vi "slow_control_2_08.vi"() -> ()   [LabVIEW 2018]
uses:
  fa57f61f-0bb9-49ac-92eb-fcb40add4dbb.vi
  499f9cf5-7b15-41ea-951a-8da9be12721d.vi
  <vilib>/DAQmx/read.llb/DAQmx Read (Analog 1D DBL NChan 1Samp).vi
  ffb0d1b3-ef19-4e2e-b36e-7277177ef4b3.vi
  9a1acc8a-69db-4048-9e4c-bb07d66d2422.vi
  <vilib>/DAQmx/create/channels.llb/DAQmx Create Channel (AI-Voltage-Basic).vi
  <vilib>/DAQmx/create/channels.llb/DAQmx Create Channel (AI-Current-Basic).vi
  <vilib>/DAQmx/create/channels.llb/DAQmx Create Channel (AI-Temperature-RTD).vi
  <vilib>/DAQmx/miscellaneous.llb/DAQmx Fill In Error Info.vi
  <vilib>/Utility/file.llb/Read Delimited Spreadsheet (string).vi
  <instrlib>/Lake Shore 335/Lake Shore 335.lvlib
  <instrlib>/CAEN PSM/CAEN PSM.lvlib
  <resource>/objmgr/daqmx.rc
panel:
  out "Cycle number":i32
  out "Alarm state":bool
  out "Timestamp last \nmeasured (UPS)":timestamp
  out "Auto-clear":bool
  in  "Auto-clear data?":bool
  in  "Clear data":bool
  in  "Clear data every N cycles":dbl
  in  "N samples":i32=30
  out "Average Flow (SLPM)":dbl caption="Flow (SLPM)"
  out "CAEN Ch. Names":string[](array[string])
  out "Heater":dbl
  out "Coldhead":dbl
  in  "Cycles to execute":dbl=5.0 format="%#_13g"
  out "Detector Pressure":dbl
  in  "N samples":i32=20
  in  "Allows tabs on \nfront panel":T1(tab)
  in  "OK Button":bool
  in  "Specify up to six temperature sensors inside \nthe detector, separated with a comma.\nNumbers only, single commas!":string="10,11,12,13,14,15"
  out "Valid example:":string="11,12, 13, 15 ,14 "
  in  "Anode ch.":enum16{"1", "2", "3", "4"}(ring)=enum."3"
  in  "CAEN unit selector":enum16{"CAEN 1", "CAEN 2"}(ring)
  in  "Multipliers":dbl[](array[numeric])=[1.0, 1.0, 1.0, 1.0, 1.0, 1.0, 1.0, 1.0]
  in  "Offsets\nsubtracted":dbl[](array[numeric])=[0.0, 0.0, 0.0, 0.0, 0.0, 0.0, 0.0, 0.0]
  in  "Channel Names (9207, ai8:15)":string[](array[string])=["i0", "i1", "i2", "i3", "i4", "i5", "i6", "i7"] caption="\"Other\""
  in  "Flow meter input:":T2(ring)=enum."v3"
  in  "Detector pressure input:":T2(ring)
  in  "Channel Names (9207, ai0:7)":string[](array[string])=["v0", "v1", "v2", "v3", "v4", "v5", "v6", "v7"] caption="\"Other\""
  in  "Multipliers":dbl[](array[numeric])=[0.2, 1.0, 1.0, 28.409091, 1.0, 1.0, 1.0, 1.0]
  in  "Offsets\nsubtracted":dbl[](array[numeric])=[0.002, 0.0, 0.0, 0.44376, 0.0, 0.0, 0.0, 0.0]
  in  "Voltage channels":tag[](array[tag])=["9207/ai0", "9207/ai1", "9207/ai2", "9207/ai3", "9207/ai4", "9207/ai5", "9207/ai6", "9207/ai7"]
  in  "COM-port CAEN 1":refnum<visa-resource-name>
  in  "COM-port CAEN 2":refnum<visa-resource-name>
  out "Temp B":dbl
  out "Temp A":dbl
  out "LakeShore readings 2":dbl[](array[numeric])
  in  "Run lakeshore?":bool
  in  "ID Query":bool
  in  "COM-port LakeShore":refnum<visa-resource-name>
  in  "PID settings":cluster{"P":dbl, "I":dbl, "D":dbl}={"P"=50.0, "I"=20.0, "D"=120.0}
  in  "Setpoint (°C)":dbl=-100.0 format="%.1f"
  in  "Heater range":u16(ring) items=["Off", "Low (On)", "Medium", "High"]
  in  "Current channels":tag[](array[tag])=["9207/ai8", "9207/ai9", "9207/ai10", "9207/ai11", "9207/ai12", "9207/ai13", "9207/ai14", "9207/ai15"]
  in  "Channel Names (CAEN)":string[](array[string])=["PMT 1", "PMT 2", "Anode", "Cathode", "Top gate", "Bottom gate", "Other 1", "Other 2"]
  in  "RTD Type":i32(ring)=12481 items=["Pt3750"=12481, "Pt3851"=10071, "Pt3911"=12482, "Pt3916"=10069, "Pt3920"=10053, "Pt3928"=12483, "Custom"=10137]
  in  "Module 1 channels (slot 1)":tag[](array[tag])
  in  "Current Excitation Source":i32(ring)=10200 items=["Internal"=10200, "External"=10167, "None"=10230]
  in  "Resistance Configuration":i32(ring)=3 items=["2-Wire"=2, "3-Wire"=3, "4-Wire"=4]
  in  "R (T = 0°C):":dbl=100.0
  in  "B":dbl
  in  "A":dbl
  in  "C":dbl
  in  "Module 2 channels (slot 2)":tag[](array[tag])
  in  "Shut off heater \nif Alarm is active":bool=TRUE
  out "Det. T.":i32[](array[numeric])
  out "9207 (V; A) Converted":dbl[](array[numeric])
  out "9216 #1 (°C)":dbl[](array[numeric])
  out "9216 #2 (°C)":dbl[](array[numeric])
  out "Raw readouts (V, mA)":dbl[](array[numeric]) format="%0.2f"
  out "Det.P input #":i32
  out "Flow input #":i32
  out "Temperatures":dbl[](array[numeric]) format="%0.2f"
  in  "Number of Bonus lines":i32=1
  out "Names (optional)":string[](array[string])
  in  "Send daily email?":bool
  in  "Phone numbers":string[](array[string])
  out "Alarm (or test) message":string
  in  "Alarm armed":bool
  in  "Repeat Alarm SMS\nevery N minutes":dbl=15.0
  in  "Test alarm":bool
  out "Warning":bool
  in  "UPS":bool
  in  "UPS Voltage \nLower Threshold":dbl=220.0
  out "String 6":string
  out "String 5":string
  out "String 4":string
  out "String 3":string
  out "String 2":string
  out "String":string
  out "NI mod 2&3 status":bool
  in  "NI mod 2&3":bool
  in  "NI mod 1":bool
  in  "CAEN 2":bool
  in  "CAEN 1":bool
  in  "LakeShore":bool
  out "Det. P. warning":bool
  out "Boolean 6":bool
  out "Boolean 5":bool
  out "Boolean 4":bool
  out "Boolean 3":bool
  out "Boolean 2":bool
  out "Boolean":bool
  in  "T 6":bool
  in  "T 5":bool
  in  "T 4":bool
  in  "T 3":bool
  in  "T 2":bool
  in  "T 1":bool
  in  "Detector Pressure":bool
  in  "Overpressure threshold":dbl
  in  "Underpressure threshold":dbl
  out "Comm. status":bool
  in  "High Temp threshold":dbl format="%#_13g"
  in  "Low Temp threshold":dbl format="%#_13g"
  out "LakeShore status":bool
  out "NI mod1 (P) status":bool
  out "CAEN 1 status":bool
  out "CAEN 2 status":bool
  out "Initialization status":bool
  out "Minimum input voltage measured":dbl
  out "Alarm active 2":bool
  out "standard error (SMS script)":string
  out "Status email preview":string
  in  "Send status email at time:":string
  in  "Email Adresses":string[](array[string])
  in  "return address":string="xamsups@gmail.com"
  in  "Ignore Initialization Errors":bool=TRUE caption="Ignore init. errors?"
  out "9207 (ai 8:15, Amperes)":cluster{timestamp[], dbl[]}[](graph)
  in  "Temperature channel selector":u16(ring)=10 items=["10"=10, "11"=11, "12"=12, "13"=13, "14"=14, "15"=15, "Average"=666]
  out "Heater power (%)":cluster{timestamp[], dbl[]}[](graph)
  out "Flow (SLPM)":cluster{timestamp[], dbl[]}[](graph)
  out "9207 (ai 0:7, Volts)":cluster{timestamp[], dbl[]}[](graph)
  out "Phase Diagram":cluster{"X":dbl, "Y":dbl}[](graph)
  out "Temperature (ai 0:15, °C)":cluster{timestamp[], dbl[]}[](graph)
  in  "Pause?":bool
  out "Integrated Flow (SL)":dbl
  in  "Reset?":bool
  out "LakeShore readings":dbl[](array[numeric])
  in  "Temperature Channel Selector":u16(ring) items=["10"=10, "11"=11, "12"=12, "13"=13, "14"=14, "15"=15]
  out "Historical Large Phase Diagram":cluster{dbl[], dbl[]}[](graph)
  out "Large Phase Diagram":cluster{"X":dbl, "Y":dbl}[](graph)
  in  "Temperature Channel Selector":u16(ring)=666 items=["10"=10, "11"=11, "12"=12, "13"=13, "14"=14, "15"=15, "Average"=666]
  in  "Scale.Range:Minimum 8":dbl
  in  "Scale.Range:Maximum 8":dbl=4000.0
  in  "Scale.Range:Minimum 7":dbl
  in  "Scale.Range:Maximum 7":dbl=4000.0
  in  "Scale.Range:Minimum 6":dbl=-3000.0
  in  "Scale.Range:Maximum 6":dbl
  in  "Scale.Range:Minimum 5":dbl
  in  "Scale.Range:Maximum 5":dbl=3000.0
  in  "Scale.Range:Minimum 4":dbl=-5000.0
  in  "Scale.Range:Maximum 4":dbl
  in  "Scale.Range:Maximum 3":dbl=4000.0
  in  "Scale.Range:Minimum 3":dbl
  in  "Scale.Range:Maximum 2":dbl=1000.0
  in  "Scale.Range:Minimum 2":dbl
  out "CAEN 1.1":dbl(knob) scale=0.0..1000.0
  out "CAEN 1.1":string
  in  "Scale.Range:Maximum":dbl=1000.0
  in  "Scale.Range:Minimum":dbl
  out "CAEN 2.3 2":string
  out "CAEN 2.2 2":string
  out "Channel Names":string[](array[string])
  out "CAEN 2.3":dbl(knob) scale=0.0..4000.0
  out "CAEN 2.2":dbl(knob) scale=0.0..4000.0
  out "CAEN 2.1":string
  out "CAEN 2.0":string
  out "CAEN 1.3":string
  out "CAEN 1.2":string
  out "CAEN 1.0":string
  out "Channel Names":string[](array[string])
  in  "Set to zero":bool
  out "CAEN 2.1":dbl(knob)
  out "CAEN 2.0":dbl(knob) scale=0.0..3000.0
  in  "Apply Voltage":bool
  in  "VSet (V)":dbl[](array[numeric])
  in  "IMax (uA)":dbl[](array[numeric])
  in  "VMax (V)":dbl[](array[numeric])
  out "CAEN 1.3":dbl(knob)
  out "CAEN 1.2":dbl(knob) scale=0.0..4000.0
  out "CAEN 1.0":dbl(knob) scale=0.0..1000.0
  out "Vmon (V)":dbl[](array[numeric])
  out "IMon (uA)":dbl[](array[numeric])
  in  "Read CAEN units \nevery N cycles":i16=120
  in  "Reset anode\nperiodically?":bool
  in  "Kill every Y minutes":i32=10
  in  "Keep off for X seconds":i32=10
  out "?":bool
  out "Killed":bool
  out "Restarted":bool
  out "Anode timers":timestamp[](array[timestamp])
  out "Seconds until \nanode autokill":dbl format="%.2g"
  out "Seconds until \nanode reset":dbl format="%.2g"
  in  "Kill voltage":bool
  in  "stop":bool
  out "Voltages":dbl[](array[numeric])
  out "Started up?":bool
  out "TOBA appended":dbl[][](array[numeric])
  in  "Read T every N cycles":i32=2
  out "Time until next cycle":dbl format="%.3g"
  in  "Time per cycle (s)":i32=2 caption="Time Target (s)"
  # "<- Proof of concept for New/Old T + New P"
  # "Moving averages"
  # "NI 9216 Temperature settings"
  # "NI 9207 Voltage settings"
  # "CAEN settings"
  # "If RTD type is custom,\nspecify the Callendar-\nVan Dusen parameters"
  # "Anode connected to:"
  # "Channel:"
  # "Lakeshore settings"
  # "NI 9207 Current settings"
  # "Brum hier"
  # "Gain (P) (XX.X)"
  # "Reset (I) (XX.X)"
  # "Rate (D) (X.X%)"
  # "Move to Quick Temp tab ^"
  # "Alarm indicators and arms"
  # "Thresholds"
  # "Daily status email"
  # "SMS and sound alarm"
  # "Alarm conditions"
  # "Uninterruptable Power Supply"
  # "Data"
  # "Scale:"
  # "to"
  # "to"
  # "Scale:"
  # "Time of last reset"
  # "Time of last reactivation"
  # "to"
  # "Scale:"
  # "to"
  # "Scale:"
  # "Settings"
  # "Scale:"
  # "to"
  # "Scale:"
  # "to"
  # "Scale:"
  # "to"
  # "to"
  # "Scale:"
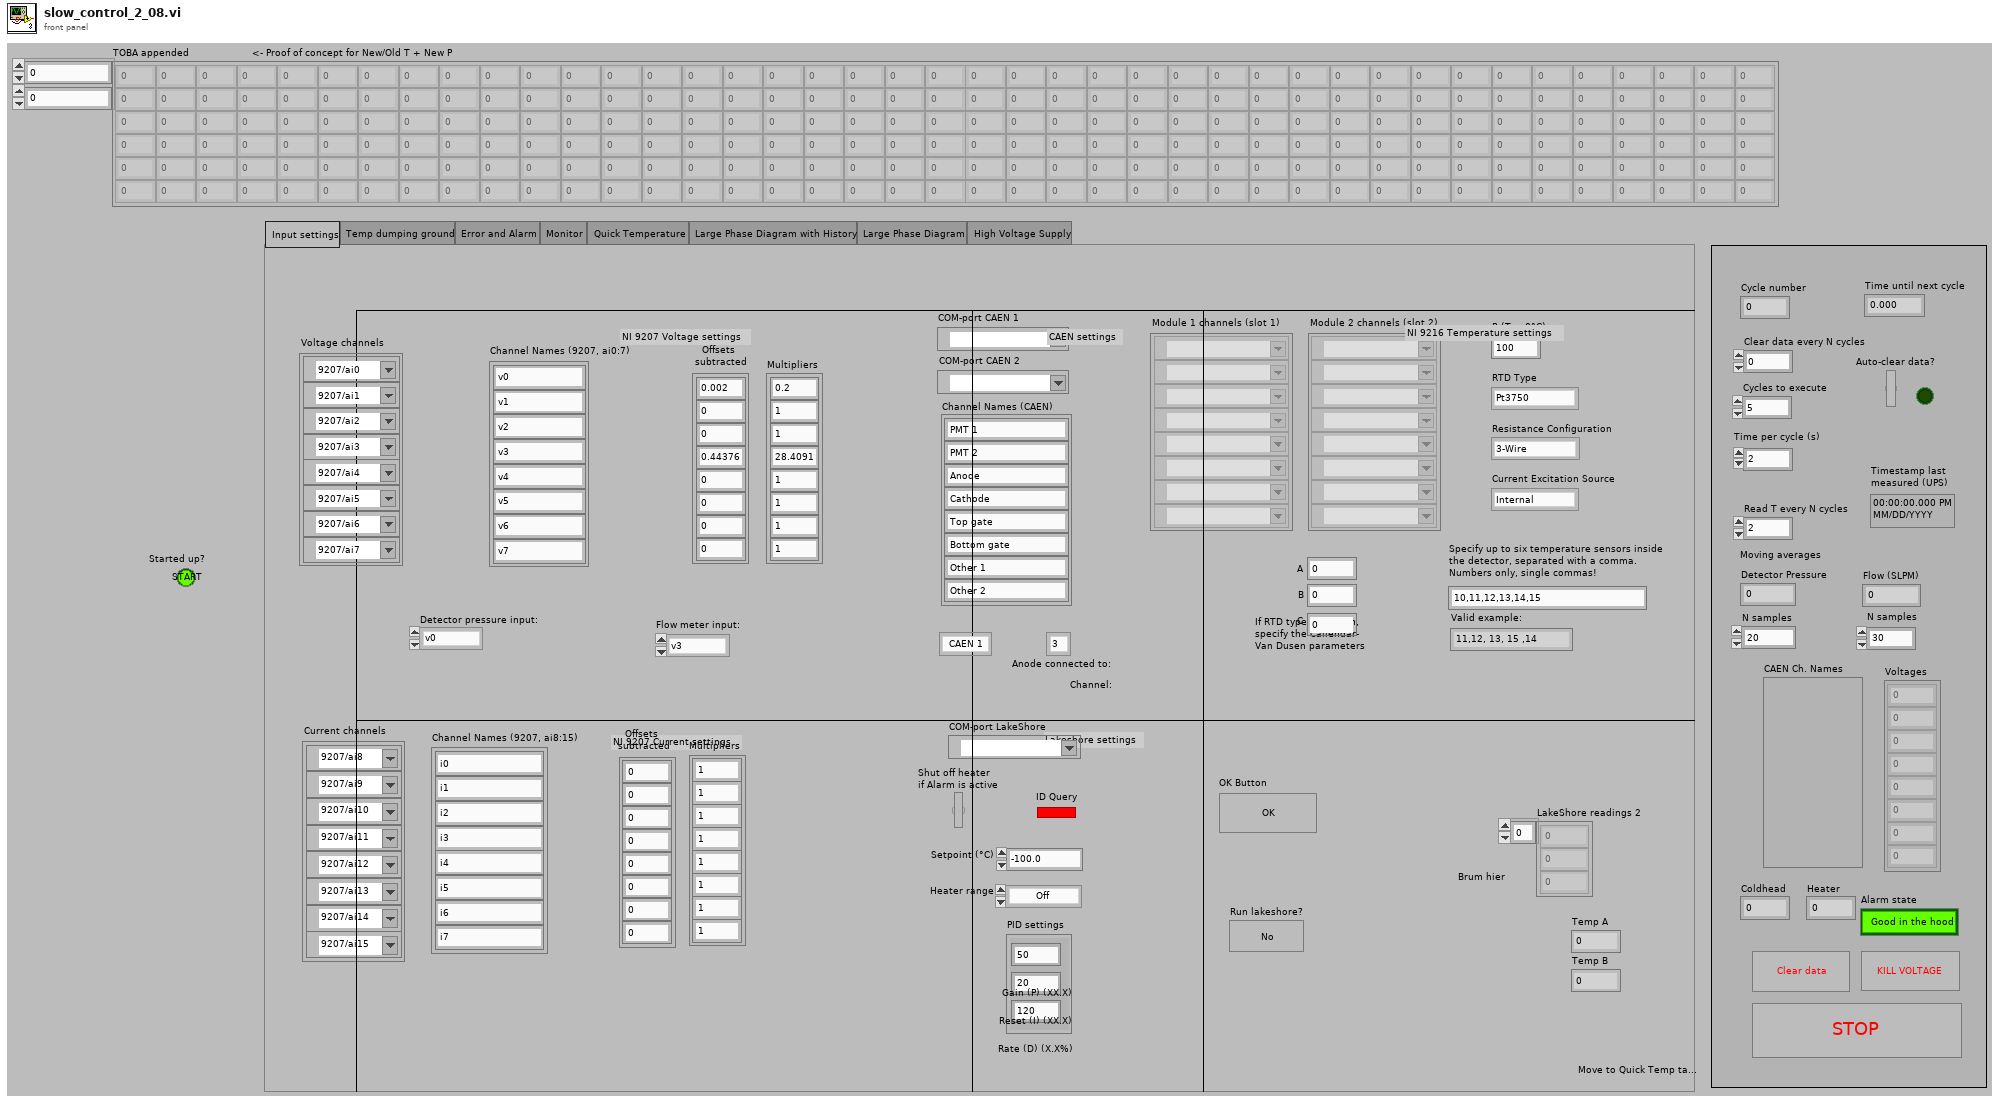
[diagram p1: front panel]
types:
  T1 = enum32{"Input settings", "Temp dumping ground", "Error and Alarm", "Monitor", "Quick Temperature", "Large Phase Diagram with History", "Large Phase Diagram", "High Voltage Supply"}
  T2 = enum16{"v0", "v1", "v2", "v3", "v4", "v5", "v6", "v7"}
  T3 = cluster{"Baud Rate":u32, "Parity":u16, "Data Bits":u16, "Stop Bits":u16, "Flow Control":u16}
  T4 = cluster{"VISA resource name out":refnum<visa-resource-name>, "error out":errorcluster}
  T5 = cluster{"task out":refnum<k21>, "error out":errorcluster}
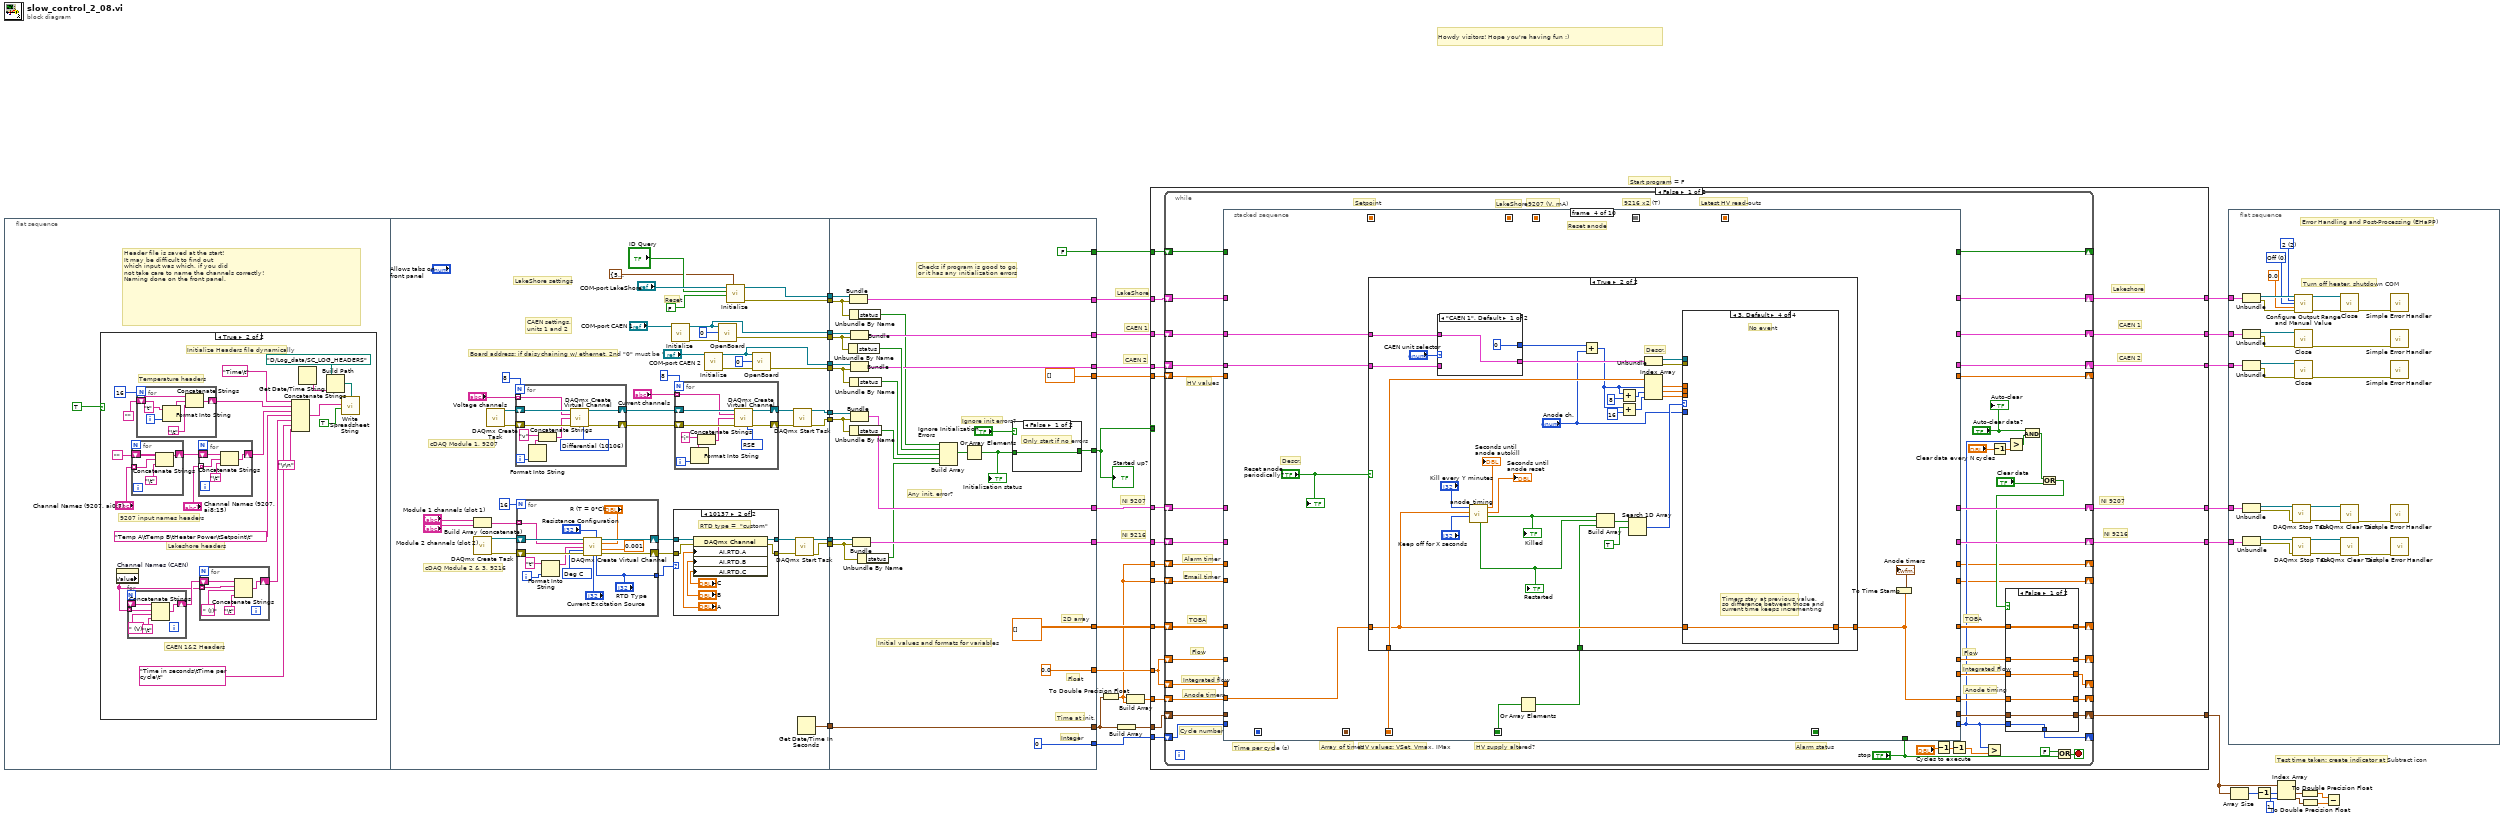
[diagram p0: block diagram]
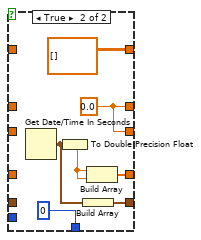
[diagram p2: hidden frame]
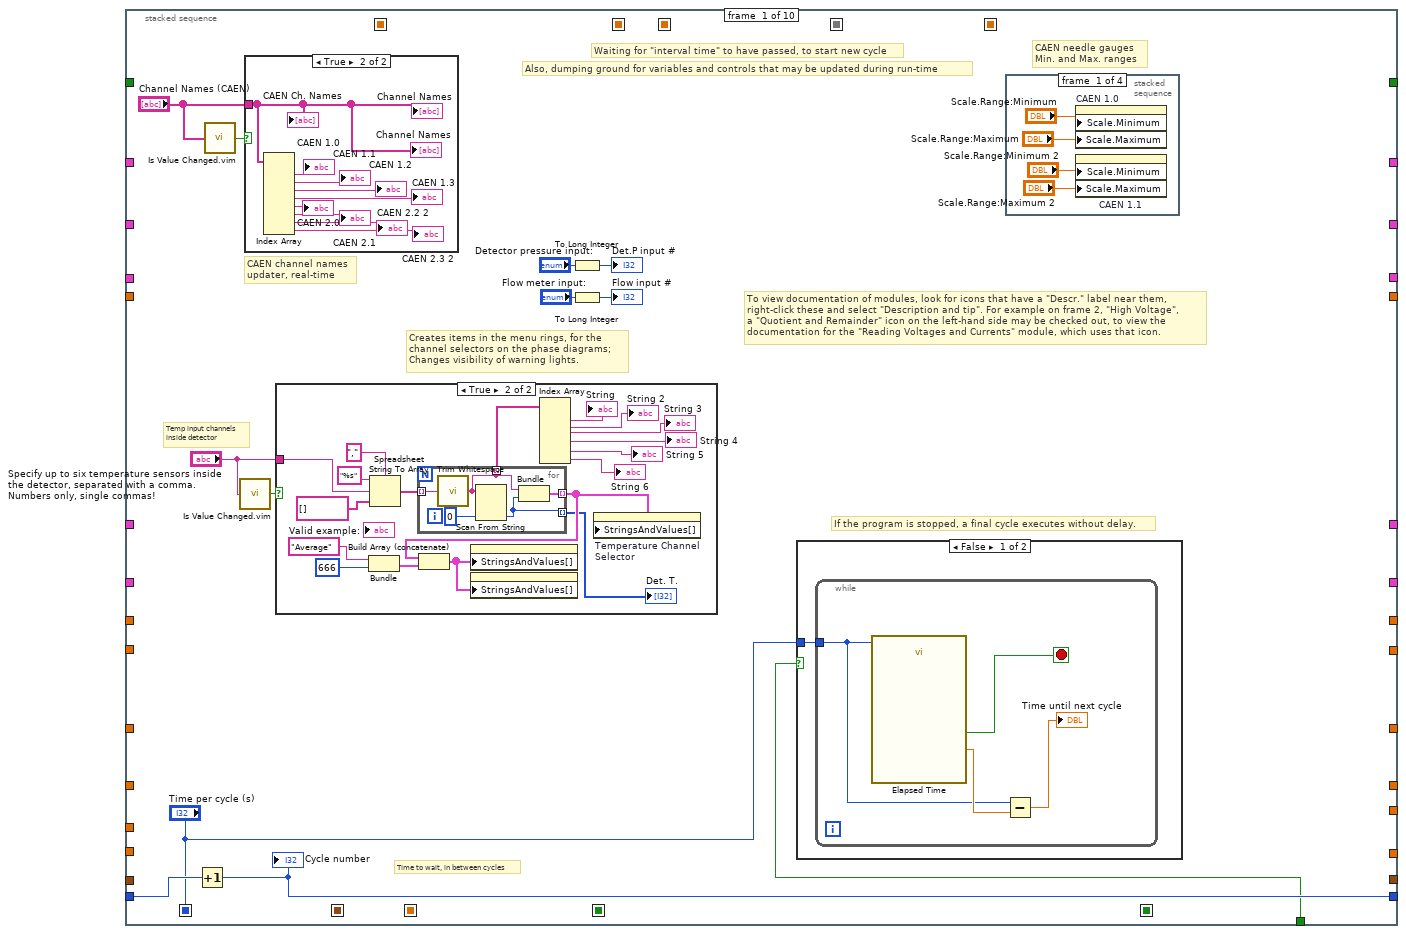
[diagram p3: hidden frame]
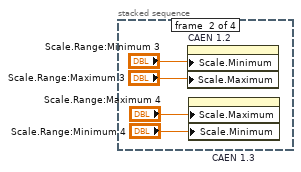
[diagram p6: hidden frame]
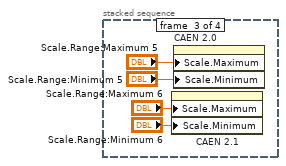
[diagram p7: hidden frame]
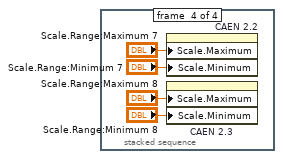
[diagram p8: hidden frame]
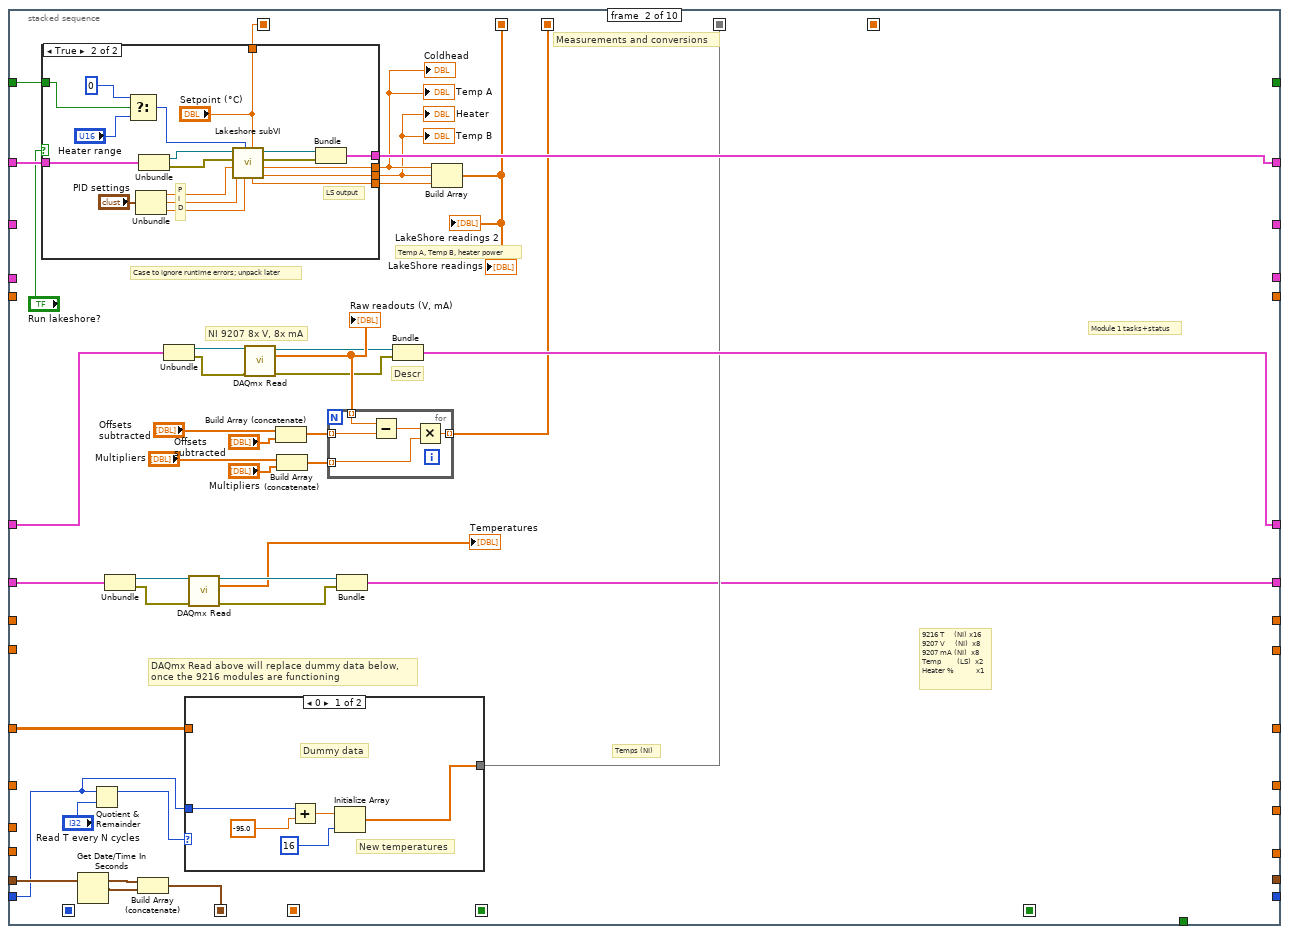
[diagram p10: hidden frame]
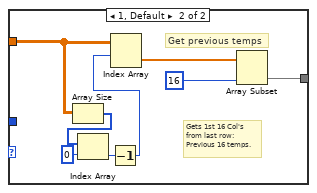
[diagram p11: hidden frame]
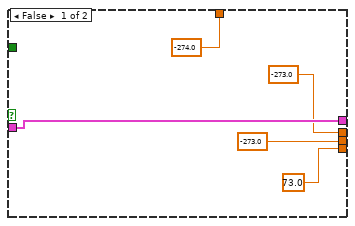
[diagram p12: hidden frame]
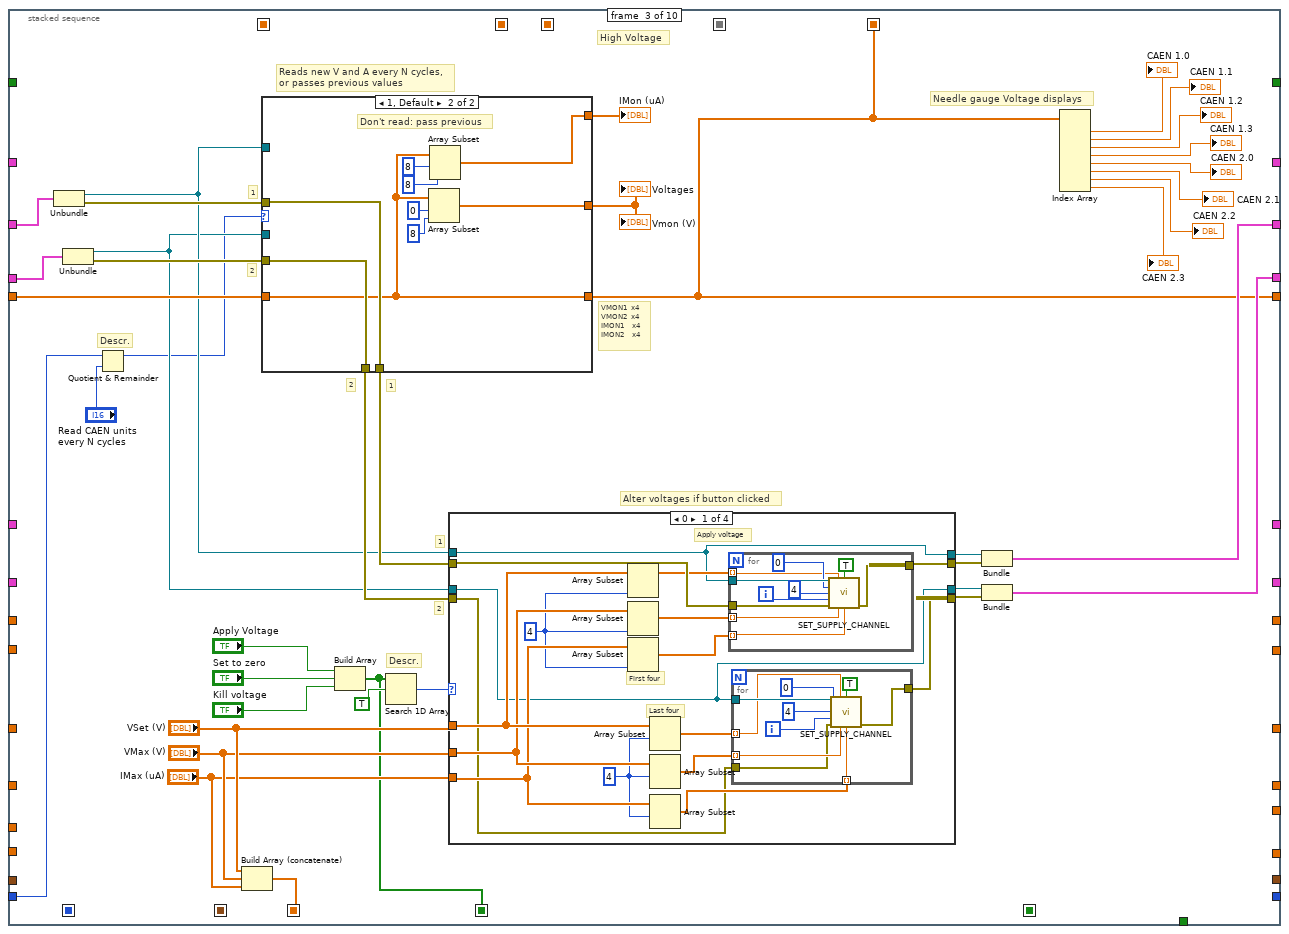
[diagram p13: hidden frame]
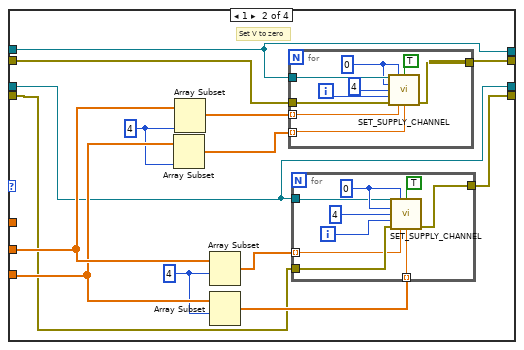
[diagram p14: hidden frame]
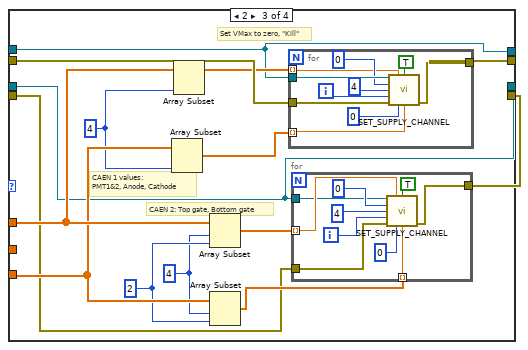
[diagram p15: hidden frame]
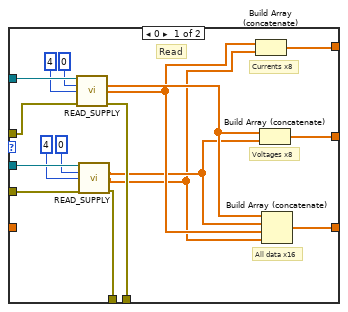
[diagram p17: hidden frame]
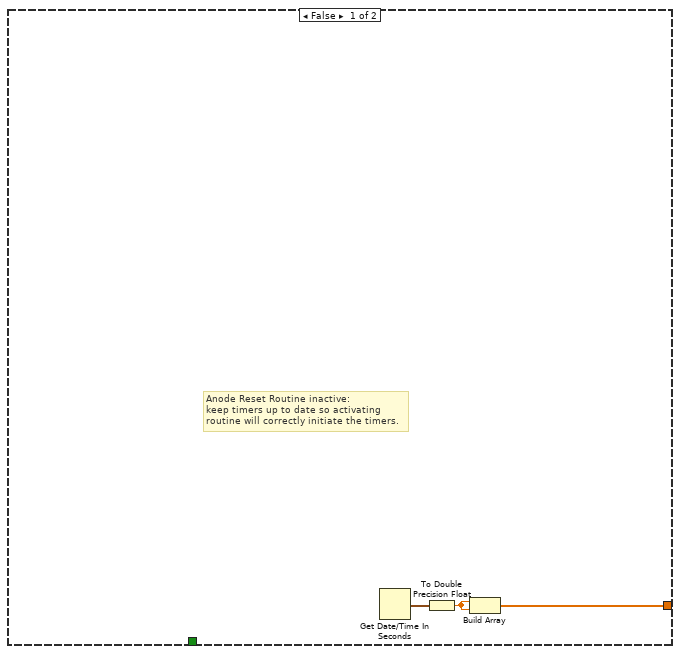
[diagram p18: hidden frame]
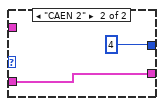
[diagram p19: hidden frame]
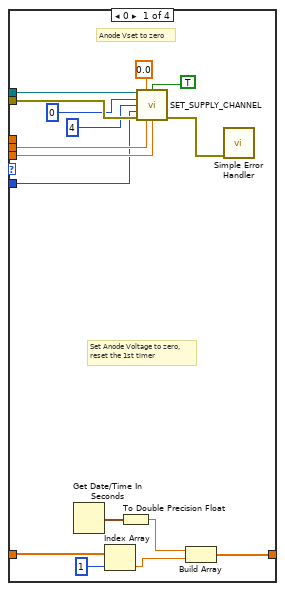
[diagram p20: hidden frame]
diagram:
  # "Howdy visitors! Hope you're having fun :)"
  # "NI 9216"
  # "Test time taken: create indicator at Subtract icon"
  # "NI 9207"
  # "Start program = F"
  # "CAEN 2"
  # "CAEN 1"
  # "LakeShore"
  n1 = flat-sequence {
    tunnel: [w123] -> w39
    tunnel: [w122] -> w38
    tunnel: [w110] -> w37
    tunnel: [w119] -> w36
    tunnel: [w100] -> w35
    tunnel: [w118] -> w30
    tunnel: [w114] -> w22
    tunnel: [w113] -> w21
    tunnel: [w101] -> w13
    tunnel: [w95] -> w5
    tunnel: [w94] -> w4
    tunnel: w39 -> [w196]
    tunnel: w38 -> [w195]
    tunnel: w37 -> [w193]
    tunnel: w36 -> [w192]
    tunnel: w35 -> [w182]
    tunnel: [w197] -> w19
    tunnel: [0.0] -> w18
    tunnel: [dbl[] []] -> w34
    tunnel: [dbl[][] []] -> w6
    tunnel: [0] -> w33
    tunnel: [w194] -> w32
    tunnel: [w191] -> w31
    tunnel: [w190] -> w17
    tunnel: w30 -> [w190]
    tunnel: w22 -> [w188]
    tunnel: w21 -> [w187]
    tunnel: [w186] -> w20
    tunnel: [FALSE] -> w14
    tunnel: w13 -> [w183]
    tunnel: [w181] -> w12
    tunnel: w5 -> [w174]
    tunnel: w4 -> [w173]
    tunnel: [w172] -> w3
    frame #0 {
      # "Header file is saved at the start!\nIt may be difficult to find out\nwhich input was which, if you did\nnot take care to name the channels correctly!\nNaming done on the front panel."
      n2 = case shown="True" TRUE {
        frame False {
        }
        frame True {
          # "CAEN 1&2 Headers"
          # "Lakeshore headers"
          # "9207 input names headers"
          # "Temperature headers"
          # "Initialize Headers file dynamically"
          n3 = property on="Channel Names (CAEN)" class="Arr (strict)"() -> ("Value"=w45:string[])  [unwired: 2 in, 2 out]
          n4 = for {
            tunnel: w45 -> [w69] mode=indexing
            shift-right: [w67] -> w46
            shift-left: _ -> [w66]
            n5 = Concatenate Strings(w66, w69, " (V)", "\t") -> (w67:string)
          }
          n6 = for {
            shift-right: [w77] -> w49
            shift-left: "" -> [w78]
            tunnel: "Channel Names (9207, ai0:7)" -> [w75] mode=indexing
            n7 = Concatenate Strings(w78, w75, "\t") -> (w77:string)
          }
          n8 = for {
            N: 16 -> [_]
            shift-right: [w79] -> w52
            shift-left: "" -> [w80]
            i -> [w84]
            n9 = Format Into String(initial string="t", w84) -> (resulting string=w82:string)  [unwired: 2 in, 1 out]
            n10 = Concatenate Strings(w80, w82, "\t") -> (w79:string)
          }
          n11 = for {
            shift-right: [w72] -> w48
            shift-left: w49 -> [w74]
            tunnel: "Channel Names (9207, ai8:15)" -> [w71] mode=indexing
            n12 = Concatenate Strings(w74, w71, "\t") -> (w72:string)
          }
          n13 = for {
            shift-right: [w62] -> w44
            shift-left: w46 -> [w63]
            tunnel: w45 -> [w61] mode=indexing
            n14 = Concatenate Strings(w63, w61, " (I)", "\t") -> (w62:string)
          }
          n15 = Concatenate Strings("Time\t", w52, w48, "Temp A\tTemp B\tHeater Power\tSetpoint\t", w44, "Time in seconds\tTime per cycle\t", "\r\n") -> (w51:string)
          n16 = Get Date/Time String() -> (date string=w55:string)  [unwired: 3 in, 1 out]
          n17 = Build Path(base path=path "D:/Log_data/SC_LOG_HEADERS" ("file path (dialog if empty)"), name or relative path=w55) -> (appended path=w56:path)
          n18 = call <vilib>:"Write Spreadsheet String.vi"("append to file? (new file:F)"=TRUE, "spreadsheet string"=w51, "file path (dialog if empty)"=w56) -> ()  [unwired: 7 in, 2 out]
        }
      }
    }
    frame #1 {
      # "cDAQ Module 2 & 3, 9216"
      # "cDAQ Module 1, 9207"
      # "Board address: if daisychaining w/ ethernet, 2nd \"0\" must be \"1\""
      # "CAEN settings,\nunits 1 and 2"
      # "Reset"
      # "LakeShore settings"
      n19 = call <vilib>:"DAQmx Create Task.vi"() -> ("task out"=w93:refnum<k21>, "error out"=w96:errorcluster)  [unwired: 14 in]
      n20 = Build Array (concatenate)("Module 1 channels (slot 1)", "Module 2 channels (slot 2)") -> (w90:tag[])
      n21 = call <vilib>:"DAQmx Create Task.vi"() -> ("task out"=w109:refnum<k21>, "error out"=w108:errorcluster)  [unwired: 14 in]
      n22 = for {
        N: 8 -> [_]
        shift-right: [w165] -> w105
        shift-left: w109 -> [w164]
        shift-right: [w166] -> w104
        shift-left: w108 -> [w162]
        tunnel: "Voltage channels" -> [w163] mode=indexing
        i -> [w168]
        w160 = 10106 items=["Default"=-1, "RSE"=10083, "NRSE"=10078, "Differential"=10106, "Pseudodifferential"=12529] ("input terminal configuration")
        n23 = Format Into String(w168) -> (resulting string=w167:string)  [unwired: 3 in, 1 out]
        n24 = Concatenate Strings("v" ("string"), w167) -> (w161:string)
        n25 = call-poly <vilib>:"DAQmx Create Virtual Channel.vi"("task in"=w164, "input terminal configuration"=w160, "physical channels"=w163, "name to assign"=w161, "error in"=w162) -> ("task out"=w165:refnum<k21>, "error out"=w166:errorcluster)  [unwired: 9 in]
      }
      n26 = for {
        N: 16 -> [_]
        shift-right: [w146] -> w89
        shift-left: w93 -> [w149]
        shift-right: [w147] -> w88
        shift-left: w96 -> [w148]
        tunnel: w90 -> [w145] mode=indexing
        tunnel: ["RTD Type"] -> w85
        i -> [w143]
        w140 = 10143 items=["Deg C"=10143, "Deg F"=10144, "Kelvins"=10325, "Deg R"=10145, "From Custom Scale"=10065] ("units")
        n27 = Format Into String(initial string="t", w143) -> (resulting string=w142:string)  [unwired: 2 in, 1 out]
        n28 = call-poly <vilib>:"DAQmx Create Virtual Channel.vi"("task in"=w149, "resistance configuration"="Resistance Configuration", "physical channels"=w145, "r0"="R (T = 0°C):", "name to assign"=w142, "units"=w140, "current excitation value"=0.001, "error in"=w148, "current excitation source"="Current Excitation Source", "rtd type"="RTD Type") -> ("task out"=w146:refnum<k21>, "error out"=w147:errorcluster)  [unwired: 4 in]
      }
      n29 = call <instrlib>:"Initialize.vi"("VISA resource name"="COM-port CAEN 1") -> ("error out"=w120:errorcluster, "VISA resource name out"=w110:refnum<visa-resource-name>)  [unwired: 9 in]
      n30 = case shown="10137" w85 {
        tunnel: w89 -> [w128 w132]
        tunnel: w88 -> [w127 w131]
        tunnel: [w128 w130] -> w87
        tunnel: [w127 w129] -> w86
        frame 0, Default {
          # "Don't need to specify the A, B, C\nvalues if RTD type is not \"custom\""
        }
        frame 10137 {
          # "RTD type =  \"custom\""
          n31 = property class="DAQmx Channel"(reference=w132, error in=w131, "AI.RTD.A"="A", "AI.RTD.B"="B", "AI.RTD.C"="C") -> (reference out=w130:refnum<k21>, error out=w129:errorcluster)
        }
      }
      n32 = for {
        N: 8 -> [_]
        shift-right: [w151] -> w102
        shift-left: w105 -> [w158]
        shift-right: [w150] -> w103
        shift-left: w104 -> [w157]
        tunnel: "Current channels" -> [w156] mode=indexing
        i -> [w155]
        w159 = 10083 items=["default"=-1, "RSE"=10083, "NRSE"=10078, "Differential"=10106, "Pseudodifferential"=12529] ("input terminal configuration")
        n33 = Format Into String(w155) -> (resulting string=w153:string)  [unwired: 3 in, 1 out]
        n34 = Concatenate Strings("i", w153) -> (w152:string)
        n35 = call-poly <vilib>:"DAQmx Create Virtual Channel.vi"("task in"=w158, "input terminal configuration"=w159, "physical channels"=w156, "name to assign"=w152, "error in"=w157) -> ("task out"=w151:refnum<k21>, "error out"=w150:errorcluster)  [unwired: 9 in]
      }
      n36 = call <instrlib>:"Initialize.vi"("VISA resource name"="COM-port CAEN 2") -> ("error out"=w115:errorcluster, "VISA resource name out"=w114:refnum<visa-resource-name>)  [unwired: 9 in]
      n37 = call <instrlib>:"OpenBoard.vi"("error in (no error)"=w120, "Board Address"=0, "VISA resource name"=w110) -> ("error out"=w119:errorcluster)  [unwired: 7 in, 1 out]
      n38 = call <instrlib>:"Initialize.vi"("Serial Configuration"=T3 {"Baud Rate"=57600, "Parity"=1, "Data Bits"=7, "Stop Bits"=10, "Flow Control"=0}, "Reset (True)"=FALSE ("Reset (LakeShore)"), "ID Query (True)"="ID Query", "VISA resource name"="COM-port LakeShore") -> ("error out"=w122:errorcluster, "VISA resource name out"=w123:refnum<visa-resource-name>)  [unwired: 6 in]
      n39 = call <instrlib>:"OpenBoard.vi"("error in (no error)"=w115, "Board Address"=u8 0, "VISA resource name"=w114) -> ("error out"=w113:errorcluster)  [unwired: 7 in, 1 out]
      n40 = call <vilib>:"DAQmx Start Task.vi"("task/channels in"=w102, "error in"=w103) -> ("task out"=w101:refnum<k21>, "error out"=w100:errorcluster)  [unwired: 12 in]
      n41 = call <vilib>:"DAQmx Start Task.vi"("task/channels in"=w87, "error in"=w86) -> ("task out"=w95:refnum<k21>, "error out"=w94:errorcluster)  [unwired: 12 in]
      n42 = Get Date/Time In Seconds() -> (seconds since 1Jan1904=w118:timestamp)
    }
    frame #2 {
      # "Initial values and formats for variables"
      # "Time at init."
      # "Integer"
      # "2D array"
      # "Float"
      # "Checks if program is good to go,\nor it has any initialization errors"
      # "Ignore init errors?"
      # "Any init. error?"
      n43 = Unbundle By Name(w192) -> ("status"=w198:bool)
      n44 = Unbundle By Name(w195) -> ("status"=w175:bool)
      n45 = Bundle("VISA resource name out"=w196, "error out"=w195) -> (w194:T4)  [unwired: 1 in]
      n46 = Unbundle By Name(w187) -> ("status"=w189:bool)
      n47 = Unbundle By Name(w182) -> ("status"=w176:bool)
      n48 = Bundle("VISA resource name out"=w188, "error out"=w187) -> (w186:T4)  [unwired: 1 in]
      n49 = Bundle("task out"=w183, "error out"=w182) -> (w181:T5)  [unwired: 1 in]
      n50 = Bundle("VISA resource name out"=w193, "error out"=w192) -> (w191:T4)  [unwired: 1 in]
      n51 = Bundle("task out"=w174, "error out"=w173) -> (w172:T5)  [unwired: 1 in]
      n52 = Unbundle By Name(w173) -> ("status"=w171:bool)
      n53 = Build Array(w175, w198, w176, w189, w171) -> (w199:bool[])
      n54 = Or Array Elements(Boolean array=w199) -> (logical OR=w170:bool)
      "Initialization status" <- w170
      n55 = case shown="False" "Ignore Initialization Errors" {
        tunnel: [w200 FALSE] -> w197
        tunnel: w170 -> [w200 _]
        frame False {
          # "Only start if no errors"
        }
        frame True {
          # "Always start program"
        }
      }
    }
  }
  n56 = To Double Precision Float(number=w17) -> (double precision float=w1:dbl)
  n57 = Build Array(w17) -> (w29:timestamp[])
  n58 = Build Array(w1, w1) -> (w16:dbl[])
  n59 = case shown="False" w19 {
    selector: w19 -> [_ w1059]
    tunnel: [_ w1059] -> _
    tunnel: w34 -> [w214 _]
    tunnel: w33 -> [w221 _]
    tunnel: w6 -> [w220 _]
    tunnel: w32 -> [w215 w1057]
    tunnel: w31 -> [w217 w1056]
    tunnel: w29 -> [w219 _]
    tunnel: [w218 timestamp[] []] -> w25
    tunnel: w20 -> [w216 w1055]
    tunnel: w18 -> [w210 _]
    tunnel: w16 -> [w213 _]
    tunnel: [w212 w1057] -> w15
    tunnel: w14 -> [w211 _]
    tunnel: w12 -> [w209 w1054]
    tunnel: [w208 w1056] -> w11
    tunnel: [w207 w1055] -> w10
    tunnel: [w206 w1054] -> w9
    tunnel: w3 -> [w205 w1053]
    tunnel: [w204 w1053] -> w2
    tunnel: w1 -> [w203 _]
    tunnel: w1 -> [w202 _]
    frame False {
      # "NI 9216"
      # "NI 9207"
      # "CAEN 2"
      # "CAEN 1"
      # "Lakeshore"
      n60 = while {
        shift-right: [w232] -> _
        shift-left: w221 -> [w270]
        shift-right: [w245] -> _
        shift-left: w220 -> [w259]
        shift-right: [w237] -> w218
        shift-left: w219 -> [w267]
        shift-right: [w261] -> w208
        shift-left: w217 -> [w254]
        shift-right: [w263] -> _
        shift-left: w214 -> [w266]
        shift-right: [w260] -> w207
        shift-left: w216 -> [w265]
        shift-right: [w262] -> w212
        shift-left: w215 -> [w264]
        shift-right: [w241] -> _
        shift-left: w210 -> [w256]
        shift-right: [w243] -> _
        shift-left: w210 -> [w257]
        shift-right: [w239] -> _
        shift-left: w213 -> [w255]
        shift-right: [w227] -> _
        shift-left: w211 -> [w253]
        shift-right: [w251] -> w206
        shift-left: w209 -> [w252]
        shift-right: [w249] -> w204
        shift-left: w205 -> [w250]
        shift-right: [w225] -> _
        shift-left: w203 -> [w226]
        shift-right: [w222] -> _
        shift-left: w202 -> [w223]
        stop <- w268 stop-if-true
        # "Email timer"
        # "Alarm timer"
        # "Alarm status"
        # "LakeShore"
        # "9216 x2 (T)"
        # "9207 (V, mA)"
        # "HV supply altered?"
        # "Setpoint"
        # "Anode timing"
        # "Anode timers"
        # "Integrated flow"
        # "Flow"
        # "Flow"
        # "Integrated Flow"
        # "TOBA"
        # "Array of times"
        # "Latest HV read-outs"
        # "Time per cycle (s)"
        # "Cycle number"
        # "HV values: VSet, Vmax, IMax"
        # "HV values"
        # "TOBA"
        n61 = stacked-sequence {
          seq-local: [_ _ w437 _ _ _ _ _ _ _] -> [_ _ _ w607 _ _ _ _ _ _]
          seq-local: ["Time per cycle (s)" _ _ _ _ _ _ _ _ _] -> [_ _ _ _ _ _ w805 _ _ _]
          seq-local: [_ _ w428 _ _ _ _ _ _ _] -> [_ _ _ _ _ _ w807 _ _ _]
          seq-local: [_ w381 _ _ _ _ _ _ _ _] -> [_ _ _ _ w688 w794 _ _ _ _]
          seq-local: [_ _ w431 _ _ _ _ _ _ _] -> [_ _ _ w602 _ _ _ _ _ _]
          seq-local: [_ w374 _ _ _ _ _ _ _ _] -> [_ _ _ _ _ _ w822 _ _ _]
          seq-local: [_ w369 _ _ _ _ _ _ _ _] -> [_ _ _ _ w713 w789 w809 w865 w900 w981]
          seq-local: [_ w368 _ _ _ _ _ _ _ _] -> [_ _ _ _ w704 w788 w810 w866 w899 w983]
          seq-local: [_ w356 _ _ _ _ _ _ _ _] -> [_ _ _ _ w711 w787 w808 _ _ _]
          seq-local: [_ _ _ _ _ _ _ w825 _ _] -> [_ _ _ _ _ _ _ _ w902 w982]
          tunnel: [w294 _ _ _ _ _ _ _ _ _] -> w231
          tunnel: "stop" -> [w293 _ _ _ _ _ _ _ _ _]
          tunnel: w270 -> [w295 w370 w459 _ _ _ _ _ _ _]
          tunnel: w259 -> [_ w371 _ _ w714 _ _ _ _ _]
          tunnel: [_ _ _ _ w690 _ _ _ _ _] -> w246
          tunnel: w267 -> [_ w383 _ _ _ _ _ _ _ _]
          tunnel: w254 -> [_ _ w466 w608 _ _ _ w882 _ _]
          tunnel: w266 -> [_ _ w464 _ _ _ _ _ _ _]
          tunnel: w265 -> [_ _ w463 w603 _ _ _ w881 _ _]
          tunnel: w264 -> [_ w384 _ _ _ _ _ w880 _ _]
          tunnel: [_ w385 _ _ _ _ _ _ _ _] -> w262
          tunnel: [_ _ w428 _ _ _ _ _ _ _] -> w263
          tunnel: [_ _ w445 _ _ _ _ _ _ _] -> w261
          tunnel: [_ _ w442 _ _ _ _ _ _ _] -> w260
          tunnel: [_ _ _ _ w688 _ _ _ _ _] -> w238
          tunnel: w256 -> [_ _ _ _ _ w792 _ _ _ _]
          tunnel: w257 -> [_ _ _ _ _ w793 _ _ _ _]
          tunnel: w255 -> [_ _ _ w609 _ _ _ _ _ _]
          tunnel: [_ _ _ w604 _ _ _ _ _ _] -> w240
          tunnel: w253 -> [_ w377 _ _ _ _ _ _ _ _]
          tunnel: w252 -> [_ w376 _ _ _ _ _ w879 _ _]
          tunnel: [_ w372 _ _ _ _ _ _ _ _] -> w251
          tunnel: [_ _ _ _ _ w791 _ _ _ _] -> w242
          tunnel: [_ _ _ _ _ w790 _ _ _ _] -> w244
          tunnel: w250 -> [_ w355 _ _ _ _ _ w867 _ _]
          tunnel: [_ w350 _ _ _ _ _ _ _ _] -> w249
          tunnel: [_ _ _ _ _ _ _ _ w904 _] -> w227
          tunnel: w226 -> [_ _ _ _ _ _ _ _ w898 _]
          tunnel: [_ _ _ _ _ _ _ _ w896 _] -> w225
          tunnel: w223 -> [_ _ _ _ _ _ _ _ _ w968]
          tunnel: [_ _ _ _ _ _ _ _ _ w967] -> w222
          frame #0 {
            # "Temp input channels\ninside detector"
            # "CAEN channel names\nupdater, real-time"
            # "Creates items in the menu rings, for the channel selectors on the phase diagrams;\nChanges visibility of warning lights."
            # "Also, dumping ground for variables and controls that may be updated during run-time"
            # "CAEN needle gauges\nMin. and Max. ranges"
            # "To view documentation of modules, look for icons that have a \"Descr.\" label near them,\nright-click these and select \"Description and tip\". For example on frame 2, \"High Voltage\",\na \"Quotient and Remainder\" icon on the left-hand side may be checked out, to view the\ndocumentation for the \"Reading Voltages and Currents\" module, which uses that icon."
            # "Time to wait, in between cycles"
            # "If the program is stopped, a final cycle executes without delay."
            # "Waiting for \"interval time\" to have passed, to start new cycle"
            n62 = Increment(x=w295) -> (x+1=w294:i32)
            "Cycle number" <- w294
            n63 = call "Is Value Changed.vim"("value"="Channel Names (CAEN)") -> ("changed or first call?"=w284:bool)
            n64 = call "Is Value Changed.vim"("value"="Specify up to six temperature sensors inside \nthe detector, separated with a comma.\nNumbers only, single commas!") -> ("changed or first call?"=w286:bool)
            n65 = case shown="True" w284 {
              tunnel: "Channel Names (CAEN)" -> [_ w296]
              frame False {
              }
              frame True {
                n66 = Index Array(array=w296) -> (element #1=→"CAEN 1.0":string, element #2=→"CAEN 1.1":string, element #3=→"CAEN 1.2":string, element #4=→"CAEN 1.3":string, element #5=→"CAEN 2.0":string, element #6=→"CAEN 2.1":string, element #7=→"CAEN 2.2 2":string, element #8=→"CAEN 2.3 2":string)  [unwired: 8 in]
                "CAEN Ch. Names" <- w296
                "Channel Names" <- w296
                "Channel Names" <- w296
              }
            }
            n67 = case shown="True" w286 {
              tunnel: "Specify up to six temperature sensors inside \nthe detector, separated with a comma.\nNumbers only, single commas!" -> [_ w306]
              frame False {
              }
              frame True {
                n68 = Bundle("Average", 666) -> (w312:cluster{string, i32})  [unwired: 1 in]
                n69 = Spreadsheet String To Array(delimiter (Tab)=",", format string="%s", spreadsheet string=w306, array type (2D Dbl)=string[] []) -> (array=w315:string[])
                n70 = for {
                  tunnel: w315 -> [w327] mode=indexing
                  tunnel: [w325] -> w314 mode=indexing
                  tunnel: [w324] -> w305 mode=indexing
                  tunnel: [w323] -> w316 mode=indexing
                  n71 = call <vilib>:"Trim Whitespace.vi"("string"=w327) -> ("trimmed string"=w323:string)  [unwired: 1 in]
                  n72 = Scan From String(input string=w323, default 1=0) -> (output 1=w324:i32)  [unwired: 3 in, 3 out]
                  n73 = Bundle("trimmed string"=w323, w324) -> (w325:cluster{"trimmed string":string, i32})  [unwired: 1 in]
                }
                "Det. T." <- w305
                n74 = Build Array (concatenate)(w314, w312) -> (w313:cluster{"trimmed string":string, i32}[])
                n75 = property on="Temperature channel selector" class="Ring (strict)"("StringsAndValues[]"=w313) -> ()  [unwired: 2 in, 2 out]
                n76 = property on="Temperature Channel Selector" class="Ring (strict)"("StringsAndValues[]"=w313) -> ()  [unwired: 2 in, 2 out]
                n77 = Index Array(array=w316) -> (element #1=→"String":string, element #2=→"String 2":string, element #3=→"String 3":string, element #4=→"String 4":string, element #5=→"String 5":string, element #6=→"String 6":string)  [unwired: 6 in]
                n78 = property on="Temperature Channel Selector" class="Ring (strict)"("StringsAndValues[]"=w314) -> ()  [unwired: 2 in, 2 out]
              }
            }
            n79 = To Long Integer(number="Detector pressure input:") -> (32bit integer=→"Det.P input #":i32)
            n80 = To Long Integer(number="Flow meter input:") -> (32bit integer=→"Flow input #":i32)
            n81 = case shown="False" w293 {
              tunnel: "Time per cycle (s)" -> [w344 _]
              frame False {
                n82 = while {
                  tunnel: w344 -> [w346]
                  stop <- w348 stop-if-true
                  n83 = call "Elapsed Time"("Time Target (s)"=w346) -> ("Elapsed Time (s)"=w347:dbl, "Time has Elapsed"=w348:bool)  [unwired: 11 in, 6 out]
                  n84 = Subtract(x=w346, y=w347) -> (x-y=→"Time until next cycle":dbl)
                }
              }
              frame True {
              }
            }
            n85 = stacked-sequence {
              frame #0 {
                n86 = property on="CAEN 1.0" class="Knob (strict)"("Scale.Minimum"="Scale.Range:Minimum", "Scale.Maximum"="Scale.Range:Maximum") -> ()  [unwired: 2 in, 2 out]
                n87 = property on="CAEN 1.1" class="Knob (strict)"("Scale.Minimum"="Scale.Range:Minimum 2", "Scale.Maximum"="Scale.Range:Maximum 2") -> ()  [unwired: 2 in, 2 out]
              }
              frame #1 {
                n88 = property on="CAEN 1.2" class="Knob (strict)"("Scale.Minimum"="Scale.Range:Minimum 3", "Scale.Maximum"="Scale.Range:Maximum 3") -> ()  [unwired: 2 in, 2 out]
                n89 = property on="CAEN 1.3" class="Knob (strict)"("Scale.Maximum"="Scale.Range:Maximum 4", "Scale.Minimum"="Scale.Range:Minimum 4") -> ()  [unwired: 2 in, 2 out]
              }
              frame #2 {
                n90 = property on="CAEN 2.1" class="Knob (strict)"("Scale.Maximum"="Scale.Range:Maximum 6", "Scale.Minimum"="Scale.Range:Minimum 6") -> ()  [unwired: 2 in, 2 out]
                n91 = property on="CAEN 2.0" class="Knob (strict)"("Scale.Maximum"="Scale.Range:Maximum 5", "Scale.Minimum"="Scale.Range:Minimum 5") -> ()  [unwired: 2 in, 2 out]
              }
              frame #3 {
                n92 = property on="CAEN 2.2" class="Knob (strict)"("Scale.Maximum"="Scale.Range:Maximum 7", "Scale.Minimum"="Scale.Range:Minimum 7") -> ()  [unwired: 2 in, 2 out]
                n93 = property on="CAEN 2.3" class="Knob (strict)"("Scale.Maximum"="Scale.Range:Maximum 8", "Scale.Minimum"="Scale.Range:Minimum 8") -> ()  [unwired: 2 in, 2 out]
              }
            }
          }
          frame #1 {
            # "DAQmx Read above will replace dummy data below,\nonce the 9216 modules are functioning"
            # "Descr"
            # "NI 9207 8x V, 8x mA"
            # "Case to ignore runtime errors; unpack later"
            # "Module 1 tasks+status"
            # "Temps (NI)"
            # "9216 T     (NI) x16\n9207 V     (NI)  x8\n9207 mA (NI)  x8\nTemp        (LS)  x2\nHeater %           x1"
            # "Temp A, Temp B, heater power"
            # "Measurements and conversions"
            n94 = case shown="True" "Run lakeshore?" {
              tunnel: [w408 w419] -> w385
              tunnel: w384 -> [w408 w418]
              tunnel: [-273.0 ("Input A") w417] -> w380
              tunnel: [-273.0 ("Input B") w416] -> w379
              tunnel: [73.0 ("Heater 1 (%)") w415] -> w378
              tunnel: w377 -> [_ w413]
              tunnel: [-274.0 "Setpoint (°C)"] -> w374
              frame False {
              }
              frame True {
                # "LS output"
                # "P\nI\nD"
                n95 = Select(t=0, s=w413, f="Heater range") -> (s? t:f=w410:i32)
                n96 = Unbundle("PID settings") -> ("P"=w424:dbl, "I"=w423:dbl, "D"=w422:dbl)
                n97 = Unbundle(w418) -> ("VISA resource name out"=w426:refnum<visa-resource-name>, "error out"=w425:errorcluster)
                n98 = call "Lakeshore subVI.vi"("Setpoint"="Setpoint (°C)", "Rate (D) (X.X %)"=w422, "Range"=w410, "Reset (I) (XX.X)"=w423, "Gain (P) (XX.X)"=w424, "error in (no error)"=w425, "VISA resource name"=w426) -> ("Input B"=w416:dbl, "Input A"=w417:dbl, "error out"=w420:errorcluster, "VISA resource name out"=w421:refnum<visa-resource-name>, "Heater 1 (%)"=w415:dbl)
                n99 = Bundle("VISA resource name out"=w421, "error out"=w420) -> (w419:T4)  [unwired: 1 in]
              }
            }
            "Temp A" <- w380
            "Temp B" <- w379
            "Heater" <- w379
            "Coldhead" <- w380
            n100 = Get Date/Time In Seconds() -> (seconds since 1Jan1904=w382:timestamp)
            n101 = Quotient & Remainder(x=w370, y="Read T every N cycles") -> (x-y*floor(x/y)=w373:i32)  [unwired: 1 out]
            n102 = Unbundle(w355) -> ("task out"=w354:refnum<k21>, "error out"=w353:errorcluster)
            n103 = Build Array (concatenate)(w383, w382) -> (w381:timestamp[])
            n104 = Unbundle(w376) -> ("task out"=w360:refnum<k21>, "error out"=w359:errorcluster)
            n105 = case shown="0" w373 {
              tunnel: w371 -> [_ w401]
              tunnel: [w394 w397] -> w368
              tunnel: w370 -> [w393 _]
              frame 0 {
                # "Dummy data"
                # "New temperatures"
                n106 = Add(x=w393, y=-95.0 ("element")) -> (x+y=w396:dbl)
                n107 = Initialize Array(w396, 16) -> (w394:dbl[])
              }
              frame 1, Default {
                # "Gets 1st 16 Col's\nfrom last row:\nPrevious 16 temps."
                # "Get previous temps"
                n108 = Array Size(array=w401) -> (size(s)=w403:i32[])
                n109 = Index Array(array=w403, index=0) -> (element=w404:i32)
                n110 = Decrement(x=w404) -> (x-1=w400:i32)
                n111 = Index Array(array=w401, index (row)=w400) -> (element=w399:dbl[])  [unwired: 1 in]
                n112 = Array Subset(array=w399, length=16) -> (w397:dbl[])  [unwired: 1 in]
              }
            }
            n113 = call-poly <vilib>:"DAQmx Read.vi"("task/channels in"=w354, "error in"=w353) -> ("task out"=w352:refnum<k21>, "data"=→"Temperatures":dbl[], "error out"=w351:errorcluster)  [unwired: 11 in]
            n114 = call-poly <vilib>:"DAQmx Read.vi"("task/channels in"=w360, "error in"=w359) -> ("task out"=w358:refnum<k21>, "data"=w367:dbl[], "error out"=w357:errorcluster)  [unwired: 11 in]
            "Raw readouts (V, mA)" <- w367
            n115 = Build Array (concatenate)("Offsets\nsubtracted", "Offsets\nsubtracted") -> (w361:dbl[])
            n116 = Build Array (concatenate)("Multipliers", "Multipliers") -> (w364:dbl[])
            n117 = for {
              tunnel: w361 -> [w391] mode=indexing
              tunnel: w367 -> [w390] mode=indexing
              tunnel: w364 -> [w388] mode=indexing
              tunnel: [w387] -> w369 mode=indexing
              n118 = Subtract(x=w390, y=w391) -> (x-y=w389:dbl)
              n119 = Multiply(x=w389, y=w388) -> (x*y=w387:dbl)
            }
            n120 = Bundle("task out"=w352, "error out"=w351) -> (w350:T5)  [unwired: 1 in]
            n121 = Bundle("task out"=w358, "error out"=w357) -> (w372:T5)  [unwired: 1 in]
            n122 = Build Array(w380, w379, w378) -> (w356:dbl[])
            "LakeShore readings" <- w356
            "LakeShore readings 2" <- w356
          }
          frame #2 {
            # "Alter voltages if button clicked"
            # "2"
            # "1"
            # "Descr."
            # "Descr."
            # "VMON1  x4 \nVMON2  x4\nIMON1    x4\nIMON2    x4"
            # "Needle gauge Voltage displays"
            # "1"
            # "2"
            # "1"
            # "2"
            # "Reads new V and A every N cycles,\nor passes previous values"
            # "High Voltage"
            n123 = Unbundle(w466) -> ("VISA resource name out"=w448:refnum<visa-resource-name>, "error out"=w465:errorcluster)
            n124 = Unbundle(w463) -> ("VISA resource name out"=w447:refnum<visa-resource-name>, "error out"=w462:errorcluster)
            n125 = Quotient & Remainder(x=w459, y="Read CAEN units \nevery N cycles") -> (x-y*floor(x/y)=w432:i32)  [unwired: 1 out]
            n126 = Build Array (concatenate)("VSet (V)", "VMax (V)", "IMax (uA)") -> (w437:dbl[])
            n127 = case shown="1, Default" w432 {
              tunnel: w448 -> [w591 _]
              tunnel: w465 -> [w590 w599]
              tunnel: w464 -> [_ w595]
              tunnel: w447 -> [w581 _]
              tunnel: w462 -> [w578 w600]
              tunnel: [w577 w600] -> w449
              tunnel: [w587 w599] -> w450
              tunnel: [w586 w595] -> w428
              tunnel: [w584 w596] -> w461
              tunnel: [w582 w592] -> w460
              frame 0 {
                # "All data x16"
                # "Voltages x8"
                # "Currents x8"
                # "Read"
                n128 = call "READ_SUPPLY.vi"("VISA resource name"=w591, "Board address"=u8 0, "NChannels"=u8 4, "error in (no error)"=w590) -> ("VMon values (V)"=w585:dbl[], "IMon values (uA)"=w583:dbl[], "error out"=w587:errorcluster)  [unwired: 9 in]
                n129 = call "READ_SUPPLY.vi"("VISA resource name"=w581, "Board address"=u8 0, "NChannels"=u8 4, "error in (no error)"=w578) -> ("VMon values (V)"=w576:dbl[], "IMon values (uA)"=w575:dbl[], "error out"=w577:errorcluster)  [unwired: 9 in]
                n130 = Build Array (concatenate)(w583, w575) -> (w582:dbl[])
                n131 = Build Array (concatenate)(w585, w576) -> (w584:dbl[])
                n132 = Build Array (concatenate)(w585, w576, w583, w575) -> (w586:dbl[])
              }
              frame 1, Default {
                # "Don't read: pass previous"
                n133 = Array Subset(array=w595, index=0, length=8) -> (w596:dbl[])
                n134 = Array Subset(array=w595, index=8, length=8) -> (w592:dbl[])
              }
            }
            "Voltages" <- w461
            "Vmon (V)" <- w461
            "IMon (uA)" <- w460
            n135 = Build Array("Apply Voltage", "Set to zero", "Kill voltage") -> (w431:bool[])
            n136 = Search 1D Array(1D array=w431, element=TRUE) -> (index of element=w451:i32)  [unwired: 1 in]
            n137 = case shown="0" w451 {
              tunnel: w450 -> [w483 w517 w550 w571]
              tunnel: w449 -> [w470 w507 w539 w573]
              tunnel: w448 -> [w479 w514 w547 w574]
              tunnel: w447 -> [w468 w505 w537 w572]
              tunnel: [w480 w515 w548 w571] -> w441
              tunnel: [w479 w514 w547 w574] -> w446
              tunnel: [w467 w504 w536 w573] -> w443
              tunnel: [w468 w505 w537 w572] -> w444
              tunnel: "VSet (V)" -> [w477 _ w545 _]
              tunnel: "VMax (V)" -> [w476 w512 _ _]
              tunnel: "IMax (uA)" -> [w475 w511 w544 _]
              frame 0 {
                w469 = 4 ("length")
                w474 = 4 ("length")
                # "Last four"
                # "First four"
                # "Apply voltage"
                n138 = Array Subset(array=w477, length=w474) -> (w482:dbl[])  [unwired: 1 in]
                n139 = Array Subset(array=w476, length=w474) -> (w481:dbl[])  [unwired: 1 in]
                n140 = Array Subset(array=w475, length=w474) -> (w478:dbl[])  [unwired: 1 in]
                n141 = Array Subset(array=w477, index=w469) -> (w473:dbl[])  [unwired: 1 in]
                n142 = Array Subset(array=w476, index=w469) -> (w472:dbl[])  [unwired: 1 in]
                n143 = Array Subset(array=w475, index=w469) -> (w471:dbl[])  [unwired: 1 in]
                n144 = for {
                  tunnel: w479 -> [w502]
                  tunnel: w483 -> [w501]
                  tunnel: w482 -> [w498] mode=indexing
                  tunnel: w481 -> [w496] mode=indexing
                  tunnel: w478 -> [w495] mode=indexing
                  tunnel: [w494] -> w480
                  i -> [w503]
                  n145 = call "SET_SUPPLY_CHANNEL.vi"("VISA resource name"=w502, "Voltage Level (0.0 V)"=w498, "Enable (OFF)"=TRUE, "Board address"=u8 0, "NChannels"=u8 4, "Channel (0)"=w503, "error in (no error)"=w501, "Voltage Max (0.0 V)"=w496, "Current Limit (0.00 uA)"=w495) -> ("error out"=w494:errorcluster)  [unwired: 6 in]
                }
                n146 = for {
                  tunnel: w468 -> [w493]
                  tunnel: w470 -> [w487]
                  tunnel: w473 -> [w492] mode=indexing
                  tunnel: w472 -> [w491] mode=indexing
                  tunnel: w471 -> [w490] mode=indexing
                  tunnel: [w486] -> w467
                  i -> [w489]
                  n147 = call "SET_SUPPLY_CHANNEL.vi"("VISA resource name"=w493, "Voltage Level (0.0 V)"=w492, "Enable (OFF)"=TRUE, "Board address"=u8 0, "NChannels"=u8 4, "Channel (0)"=w489, "error in (no error)"=w487, "Voltage Max (0.0 V)"=w491, "Current Limit (0.00 uA)"=w490) -> ("error out"=w486:errorcluster)  [unwired: 6 in]
                }
              }
              frame 1 {
                w506 = 4 ("length")
                w510 = 4 ("length")
                # "Set V to zero"
                n148 = Array Subset(array=w511, length=w510) -> (w513:dbl[])  [unwired: 1 in]
                n149 = Array Subset(array=w512, length=w510) -> (w516:dbl[])  [unwired: 1 in]
                n150 = Array Subset(array=w512, index=w506) -> (w509:dbl[])  [unwired: 1 in]
                n151 = Array Subset(array=w511, index=w506) -> (w508:dbl[])  [unwired: 1 in]
                n152 = for {
                  tunnel: w514 -> [w534]
                  tunnel: w517 -> [w533]
                  tunnel: w516 -> [w530] mode=indexing
                  tunnel: w513 -> [w529] mode=indexing
                  tunnel: [w528] -> w515
                  i -> [w535]
                  w527 = u8 0 ("Board address")
                  n153 = call "SET_SUPPLY_CHANNEL.vi"("VISA resource name"=w534, "Voltage Level (0.0 V)"=w527, "Enable (OFF)"=TRUE, "Board address"=w527, "NChannels"=u8 4, "Channel (0)"=w535, "error in (no error)"=w533, "Voltage Max (0.0 V)"=w530, "Current Limit (0.00 uA)"=w529) -> ("error out"=w528:errorcluster)  [unwired: 6 in]
                }
                n154 = for {
                  tunnel: w505 -> [w518]
                  tunnel: w507 -> [w523]
                  tunnel: w509 -> [w522] mode=indexing
                  tunnel: w508 -> [w521] mode=indexing
                  tunnel: [w519] -> w504
                  i -> [w524]
                  w526 = 0 ("length")
                  n155 = call "SET_SUPPLY_CHANNEL.vi"("VISA resource name"=w518, "Voltage Level (0.0 V)"=w526, "Enable (OFF)"=TRUE, "Board address"=w526, "NChannels"=u8 4, "Channel (0)"=w524, "error in (no error)"=w523, "Voltage Max (0.0 V)"=w522, "Current Limit (0.00 uA)"=w521) -> ("error out"=w519:errorcluster)  [unwired: 6 in]
                }
              }
              frame 2 {
                w538 = 4 ("length")
                w542 = 2 ("length")
                w543 = 4 ("length")
                # "CAEN 2: Top gate, Bottom gate"
                # "CAEN 1 values:\nPMT1&2, Anode, Cathode"
                # "Set VMax to zero, \"Kill\""
                n156 = Array Subset(array=w544, length=w543) -> (w546:dbl[])  [unwired: 1 in]
                n157 = Array Subset(array=w545, length=w543) -> (w549:dbl[])  [unwired: 1 in]
                n158 = Array Subset(array=w545, index=w538, length=w542) -> (w541:dbl[])
                n159 = Array Subset(array=w544, index=w538, length=w542) -> (w540:dbl[])
                n160 = for {
                  tunnel: w547 -> [w569]
                  tunnel: w550 -> [w568]
                  tunnel: w549 -> [w565] mode=indexing
                  tunnel: w546 -> [w563] mode=indexing
                  tunnel: [w562] -> w548
                  i -> [w570]
                  n161 = call "SET_SUPPLY_CHANNEL.vi"("VISA resource name"=w569, "Voltage Level (0.0 V)"=w565, "Enable (OFF)"=TRUE, "Board address"=u8 0, "NChannels"=u8 4, "Channel (0)"=w570, "error in (no error)"=w568, "Voltage Max (0.0 V)"=u8 0 ("Board address"), "Current Limit (0.00 uA)"=w563) -> ("error out"=w562:errorcluster)  [unwired: 6 in]
                }
                n162 = for {
                  tunnel: w537 -> [w551]
                  tunnel: w539 -> [w554]
                  tunnel: w541 -> [w557] mode=indexing
                  tunnel: w540 -> [w555] mode=indexing
                  tunnel: [w553] -> w536
                  i -> [w560]
                  n163 = call "SET_SUPPLY_CHANNEL.vi"("VISA resource name"=w551, "Voltage Level (0.0 V)"=w557, "Enable (OFF)"=TRUE, "Board address"=u8 0, "NChannels"=u8 4, "Channel (0)"=w560, "error in (no error)"=w554, "Voltage Max (0.0 V)"=0, "Current Limit (0.00 uA)"=w555) -> ("error out"=w553:errorcluster)  [unwired: 6 in]
                }
              }
              frame 3, Default {
                # "\"Executes\" if none of the three buttons have been clicked"
                # "Do nothing"
              }
            }
            n164 = Bundle("VISA resource name out"=w446, "error out"=w441) -> (w445:T4)  [unwired: 1 in]
            n165 = Bundle("VISA resource name out"=w444, "error out"=w443) -> (w442:T4)  [unwired: 1 in]
            n166 = Index Array(array=w428) -> (element #1=→"CAEN 1.0":dbl, element #2=→"CAEN 1.1":dbl, element #3=→"CAEN 1.2":dbl, element #4=→"CAEN 1.3":dbl, element #5=→"CAEN 2.0":dbl, element #6=→"CAEN 2.1":dbl, element #7=→"CAEN 2.2":dbl, element #8=→"CAEN 2.3":dbl)  [unwired: 8 in]
          }
          frame #3 {
            # "Descr."
            # "Reset anode"
            n167 = Or Array Elements(Boolean array=w602) -> (logical OR=w601:bool)
            n168 = case shown="True" "Reset anode\nperiodically?" {
              tunnel: w609 -> [_ w615]
              tunnel: w608 -> [_ w624]
              tunnel: w607 -> [_ w629]
              tunnel: w601 -> [_ w613]
              tunnel: [w610 w614] -> w604
              tunnel: w603 -> [_ w623]
              frame False {
                # "Anode Reset Routine inactive:\nkeep timers up to date so activating\nroutine will correctly initiate the timers."
                n169 = Get Date/Time In Seconds() -> (seconds since 1Jan1904=w612:timestamp)
                n170 = To Double Precision Float(number=w612) -> (double precision float=w611:dbl)
                n171 = Build Array(w611, w611) -> (w610:dbl[])
              }
              frame True {
                # "Descr."
                n172 = case shown="\"CAEN 1\", Default" "CAEN unit selector" {
                  tunnel: w624 -> [w643 _]
                  tunnel: w623 -> [_ w645]
                  tunnel: [w643 w645] -> w622
                  tunnel: [0 4] -> w620
                  frame "CAEN 1", Default {
                  }
                  frame "CAEN 2" {
                  }
                }
                n173 = call "anode_timing.vi"("Keep off for X seconds"="Keep off for X seconds", "Array of timers"=w615, "Kill every Y minutes"="Kill every Y minutes") -> ("Time to kill"=w631:bool, "Time until reset"=→"Seconds until \nanode reset":dbl, "Time until autokill"=→"Seconds until \nanode autokill":dbl, "Time to reset"=w632:bool)  [unwired: 5 in]
                "Killed" <- w631
                "Restarted" <- w632
                n174 = Add(x=w620, y="Anode ch.") -> (x+y=w618:i32)
                n175 = Build Array(w631, w632, w613) -> (w635:bool[])
                n176 = Add(x=w618, y=8) -> (x+y=w625:i32)
                n177 = Add(x=w618, y=16) -> (x+y=w626:i32)
                n178 = Search 1D Array(1D array=w635, element=TRUE) -> (index of element=w634:i32)  [unwired: 1 in]
                n179 = Unbundle(w622) -> ("VISA resource name out"=w640:refnum<visa-resource-name>, "error out"=w639:errorcluster)
                n180 = Index Array(array=w629, index #1=w618, index #2=w625, index #3=w626) -> (element #1=w638:dbl, element #2=w636:dbl, element #3=w637:dbl)
                n181 = case shown="3, Default" w634 {
                  tunnel: w638 -> [_ w669 _ _]
                  tunnel: w636 -> [w654 w668 _ _]
                  tunnel: w637 -> [w656 w667 _ _]
                  tunnel: w640 -> [w661 w672 _ _]
                  tunnel: w639 -> [w660 w671 _ _]
                  tunnel: "Anode ch." -> [w652 w665 _ _]
                  tunnel: w615 -> [w647 _ _ w678]
                  tunnel: [w646 w662 w675 w678] -> w614
                  frame 0 {
                    # "Set Anode Voltage to zero,\nreset the 1st timer"
                    # "Anode Vset to zero"
                    n182 = Get Date/Time In Seconds() -> (seconds since 1Jan1904=w650:timestamp)
                    n183 = Index Array(array=w647, index=1) -> (element=w648:dbl)
                    n184 = To Double Precision Float(number=w650) -> (double precision float=w649:dbl)
                    n185 = call "SET_SUPPLY_CHANNEL.vi"("VISA resource name"=w661, "Voltage Level (0.0 V)"=0.0, "Enable (OFF)"=TRUE, "Board address"=u8 0, "NChannels"=u8 4, "Channel (0)"=w652, "error in (no error)"=w660, "Voltage Max (0.0 V)"=w654, "Current Limit (0.00 uA)"=w656) -> ("error out"=w655:errorcluster)  [unwired: 6 in]
                    n186 = Build Array(w649, w648) -> (w646:dbl[])
                    n187 = call <vilib>:"Simple Error Handler.vi"("error in (no error)"=w655) -> ()  [unwired: 4 in, 5 out]
                  }
                  frame 1 {
                    # "Set Anode Voltage to defined value,\nreset both timers"
                    # "Anode Vset applied"
                    n188 = Get Date/Time In Seconds() -> (seconds since 1Jan1904=w664:timestamp)
                    n189 = To Double Precision Float(number=w664) -> (double precision float=w663:dbl)
                    n190 = call "SET_SUPPLY_CHANNEL.vi"("VISA resource name"=w672, "Voltage Level (0.0 V)"=w669, "Enable (OFF)"=TRUE, "Board address"=u8 0, "NChannels"=u8 4, "Channel (0)"=w665, "error in (no error)"=w671, "Voltage Max (0.0 V)"=w668, "Current Limit (0.00 uA)"=w667) -> ("error out"=w666:errorcluster)  [unwired: 6 in]
                    n191 = Build Array(w663, w663) -> (w662:dbl[])
                    n192 = call <vilib>:"Simple Error Handler.vi"("error in (no error)"=w666) -> ()  [unwired: 4 in, 5 out]
                  }
                  frame 2 {
                    # "Change Voltage button pressed"
                    # "Reset both timers"
                    n193 = Get Date/Time In Seconds() -> (seconds since 1Jan1904=w677:timestamp)
                    n194 = To Double Precision Float(number=w677) -> (double precision float=w676:dbl)
                    n195 = Build Array(w676, w676) -> (w675:dbl[])
                  }
                  frame 3, Default {
                    # "Timers stay at previous value,\nso difference between those and\ncurrent time keeps incrementing"
                    # "No event"
                  }
                }
              }
            }
            n196 = To Time Stamp(1:w604) -> (0:→"Anode timers":timestamp[])
            "?" <- "Reset anode\nperiodically?"
          }
          frame #4 {
            w693 = 16 ("index")
            # "Plots 9207 output vs time"
            # "Descr."
            # "Moving averages"
            # "Historic graphs: Phase, 9207 ai, Flow, Heater, Temperature"
            # "Non-historic Temperature + Det. Pressure"
            # "Updated TOBA"
            # "Descr."
            # "Latest Detector Pressure"
            # "Plots individual lists of Temp. vs. t"
            # "Plots and moving averages"
            n197 = Build Array (concatenate)(w704, w713, w711) -> (w712:dbl[])
            n198 = Build Array (concatenate)(w714, w712) -> (w690:dbl[][])
            "TOBA appended" <- w690
            n199 = local read "Det. T."() -> (w683:i32[])
            n200 = local read "Flow input #"() -> (w679:i32)
            n201 = local read "Det.P input #"() -> (w680:i32)
            n202 = Equal?(x=666, y="Temperature channel selector") -> (x = y?=w705:bool)
            n203 = Index Array(array=w690, index (col)=34 ("disabled index (col)")) -> (element=w698:dbl[])  [unwired: 1 in]
            n204 = case shown="True" w705 {
              tunnel: w704 -> [w759 w765]
              tunnel: w683 -> [_ w764]
              tunnel: [w758 w760] -> w702
              tunnel: "Temperature channel selector" -> [w757 _]
              frame False {
                n205 = Index Array(array=w759, index=w757) -> (element=w758:dbl)
              }
              frame True {
                n206 = for {
                  tunnel: w765 -> [w768]
                  tunnel: w764 -> [w767] mode=indexing
                  tunnel: [w766] -> w761 mode=indexing
                  n207 = Index Array(array=w768, index=w767) -> (element=w766:dbl)
                }
                n208 = Array Size(array=w761) -> (size(s)=w763:i32)
                n209 = Add Array Elements(numeric array=w761) -> (sum=w762:dbl)
                n210 = Divide(x=w762, y=w763) -> (x/y=w760:dbl)
              }
            }
            n211 = Add(x=w680, y=w693) -> (x+y=w695:i32)
            n212 = Add(x=w693, y=w679) -> (x+y=w692:i32)
            n213 = Index Array(array=w690, index (col) #1=w695, index (col) #2=w692) -> (element #1=w694:dbl[], element #2=w691:dbl[])  [unwired: 2 in]
            n214 = Index Array(array=w690, index (col)="Temperature Channel Selector") -> (element=w700:dbl[])  [unwired: 1 in]
            n215 = local read "Det.P input #"() -> (w681:i32)
            n216 = Bundle(w700, w694) -> (w732:cluster{dbl[], dbl[]})  [unwired: 1 in]
            n217 = for {
              N: 8 -> [_]
              tunnel: w690 -> [w749]
              tunnel: w688 -> [w741]
              tunnel: [w746] -> w687 mode=indexing
              tunnel: [w740] -> w686 mode=indexing
              i -> [w745]
              n218 = Add(x=w745, y=24) -> (x+y=w743:i32)
              n219 = Add(x=16, y=w745) -> (x+y=w748:i32)
              n220 = Index Array(array=w749, index (col) #1=w748, index (col) #2=w743) -> (element #1=w747:dbl[], element #2=w742:dbl[])  [unwired: 2 in]
              n221 = Bundle(w741, w747) -> (w746:cluster{timestamp[], dbl[]})  [unwired: 1 in]
              n222 = Bundle(w741, w742) -> (w740:cluster{timestamp[], dbl[]})  [unwired: 1 in]
            }
            "9207 (ai 0:7, Volts)" <- w687
            "9207 (ai 8:15, Amperes)" <- w686
            n223 = Bundle(w688, w691) -> (w730:cluster{timestamp[], dbl[]})  [unwired: 1 in]
            n224 = Build Array(w730) -> (→"Flow (SLPM)":cluster{timestamp[], dbl[]}[])
            n225 = Index Array(array=w713, index=w681) -> (element=w733:dbl)
            n226 = Build Array(w732) -> (→"Historical Large Phase Diagram":cluster{dbl[], dbl[]}[])
            n227 = Bundle(w702, w733) -> (w737:cluster{dbl, dbl})  [unwired: 1 in]
            n228 = Bundle(w688, w698) -> (w728:cluster{timestamp[], dbl[]})  [unwired: 1 in]
            n229 = Build Array(w728) -> (→"Heater power (%)":cluster{timestamp[], dbl[]}[])
            n230 = Build Array(w737) -> (→"Phase Diagram":cluster{dbl, dbl}[])
            n231 = Reverse 1D Array(array=w694) -> (reversed array=w727:dbl[])
            n232 = Array Subset(array=w727, length="N samples") -> (w717:dbl[])  [unwired: 1 in]
            n233 = local read "Det. T."() -> (w682:i32[])
            n234 = Array Size(array=w717) -> (size(s)=w716:i32)
            n235 = Add Array Elements(numeric array=w717) -> (sum=w726:dbl)
            n236 = Divide(x=w726, y=w716) -> (x/y=→"Detector Pressure":dbl)
            n237 = Equal?(x=666, y="Temperature Channel Selector") -> (x = y?=w707:bool)
            n238 = for {
              N: 16 -> [_]
              tunnel: w688 -> [w785]
              tunnel: [w784] -> w738 mode=indexing
              tunnel: w690 -> [w783]
              i -> [w782]
              n239 = Index Array(array=w783, index (col)=w782) -> (element=w781:dbl[])  [unwired: 1 in]
              n240 = Bundle(w785, w781) -> (w784:cluster{timestamp[], dbl[]})  [unwired: 1 in]
            }
            "Temperature (ai 0:15, °C)" <- w738
            n241 = case shown="True" w707 {
              tunnel: w704 -> [w771 w777]
              tunnel: w682 -> [_ w776]
              tunnel: [w770 w772] -> w710
              tunnel: "Temperature Channel Selector" -> [w769 _]
              frame False {
                n242 = Index Array(array=w771, index=w769) -> (element=w770:dbl)
              }
              frame True {
                n243 = for {
                  tunnel: w777 -> [w780]
                  tunnel: w776 -> [w779] mode=indexing
                  tunnel: [w778] -> w773 mode=indexing
                  n244 = Index Array(array=w780, index=w779) -> (element=w778:dbl)
                }
                n245 = Array Size(array=w773) -> (size(s)=w775:i32)
                n246 = Add Array Elements(numeric array=w773) -> (sum=w774:dbl)
                n247 = Divide(x=w774, y=w775) -> (x/y=w772:dbl)
              }
            }
            n248 = local read "Channel Names (9207, ai8:15)"() -> (w685:string[])
            n249 = local read "Channel Names (9207, ai0:7)"() -> (w684:string[])
            n250 = Reverse 1D Array(array=w691) -> (reversed array=w723:dbl[])
            n251 = Array Subset(array=w723, length="N samples") -> (w719:dbl[])  [unwired: 1 in]
            n252 = Array Size(array=w719) -> (size(s)=w718:i32)
            n253 = call "Is Value Changed.vim"("value"=w685) -> ("changed or first call?"=w696:bool)
            n254 = call "Is Value Changed.vim"("value"=w684) -> ("changed or first call?"=w697:bool)
            n255 = Add Array Elements(numeric array=w719) -> (sum=w722:dbl)
            n256 = Bundle(w710, w733) -> (w735:cluster{dbl, dbl})  [unwired: 1 in]
            n257 = Divide(x=w722, y=w718) -> (x/y=→"Average Flow (SLPM)":dbl)
            n258 = case shown="True" w696 {
              tunnel: w685 -> [_ w751]
              frame False {
              }
              frame True {
                n259 = for {
                  tunnel: w751 -> [w752] mode=indexing
                  i -> [w753]
                  n260 = property on="9207 (ai 8:15, Amperes)" class="XYGraph (strict)"("Active Plot"=w753, "Plot.Plot Name"=w752) -> ()  [unwired: 2 in, 2 out]
                }
              }
            }
            n261 = case shown="True" w697 {
              tunnel: w684 -> [_ w754]
              frame False {
              }
              frame True {
                n262 = for {
                  tunnel: w754 -> [w755] mode=indexing
                  i -> [w756]
                  n263 = property on="9207 (ai 0:7, Volts)" class="XYGraph (strict)"("Active Plot"=w756, "Plot.Plot Name"=w755) -> ()  [unwired: 2 in, 2 out]
                }
              }
            }
            n264 = Build Array(w735) -> (→"Large Phase Diagram":cluster{dbl, dbl}[])
          }
          frame #5 {
            # "Temp A, Temp B, Heater%"
            # "To indicators on the physical schematic"
            # "Separate latest 9207 readings.\nIndicators go here"
            # "Displays"
            n265 = local read "Flow input #"() -> (w786:i32)
            n266 = case shown="False" "Reset?" {
              tunnel: [w799 0.0] -> w795
              tunnel: w792 -> [w799 _]
              frame False {
              }
              frame True {
              }
            }
            n267 = Index Array(array=w789) -> ()  [unwired: 8 in, 8 out]
            n268 = Index Array(array=w789, index=w786) -> (element=w790:dbl)
            n269 = call "Average_flow_x_time.vi"("Array of timestamps"=w794, "Previous Flow"=w793, "Latest Flow"=w790) -> ("Volume (SL)"=w796:dbl)  [unwired: 8 in]
            n270 = case shown="False" "Pause?" {
              tunnel: w795 -> [w803 w804]
              tunnel: w796 -> [w802 _]
              tunnel: [w801 w804] -> w791
              frame False {
                n271 = Add(x=w802, y=w803) -> (x+y=w801:dbl)
              }
              frame True {
              }
            }
            "Integrated Flow (SL)" <- w791
            n272 = Index Array(array=w787) -> ()  [unwired: 3 in, 3 out]
            n273 = Index Array(array=w788) -> ()  [unwired: 16 in, 16 out]
            "9207 (V; A) Converted" <- w789
            "9216 #1 (°C)" <- w788
            "9216 #2 (°C)" <- w788
          }
          frame #6 {
            # "-----------DATA SAVED----------\nHuman-readable timestamp  ;\nTemperatures (16),  2xNI 9216;\nVolts, Amps  (16),       NI 9207;\nTemperature (2),    Lakeshore;\nHeater power (1),  Lakeshore;\nSetpoint (1),           Lakeshore;\nHV readouts (16)          CAEN ;\nCurrent time (s)                ---   ;\nCycle time (s)                    ---   ;"
            # "Saving data"
            n274 = Get Date/Time In Seconds() -> (seconds since 1Jan1904=w821:timestamp)
            n275 = To Double Precision Float(number=w821) -> (double precision float=w806:dbl)
            n276 = Build Array (concatenate)(w810, w809, w808, w822, w807, w806, w805) -> (w820:dbl[])
            n277 = Get Date/Time String() -> (date string=w814:string)  [unwired: 3 in, 1 out]
            n278 = Build Path(base path=path "D:/Log_data/SC_LOG", name or relative path=w814) -> (appended path=w813:path)
            n279 = Format Date/Time String() -> (date/time string=w818:string)  [unwired: 3 in]
            n280 = Array To Spreadsheet String(array=w820, 3:"%.3f" ("format string")) -> (spreadsheet string=w816:string)  [unwired: 1 in]
            n281 = Concatenate Strings(w818, "\t", w816) -> (w812:string)
            n282 = call <vilib>:"Write Spreadsheet String.vi"("append to file? (new file:F)"=TRUE, "spreadsheet string"=w812, "file path (dialog if empty)"=w813) -> ()  [unwired: 7 in, 2 out]
          }
          frame #7 {
            # "Status is True if ANY (armed)\ncondition is met"
            # "Detector P. Alert"
            # "Uninteruptable\n Power Supply Alert"
            # "Temp. Warning"
            # "Arms"
            # "Comm. Alert"
            # "Temperature Alert"
            # "Alarm conditions (Temp)"
            # "Check Alarms and Warnings"
            n283 = Unbundle By Name(w867) -> ("error out.status"=w848:bool)
            "NI mod 2&3 status" <- w848
            n284 = Unbundle By Name(w880) -> ("error out.status"=w878:bool)
            "LakeShore status" <- w878
            n285 = Unbundle By Name(w882) -> ("error out.status"=w877:bool)
            "CAEN 1 status" <- w877
            n286 = Unbundle By Name(w881) -> ("error out.status"=w876:bool)
            "CAEN 2 status" <- w876
            n287 = Unbundle By Name(w879) -> ("error out.status"=w875:bool)
            "NI mod1 (P) status" <- w875
            n288 = Build Array(w878, w877, w876, w875, w848) -> (w849:bool[])
            n289 = Build Array("LakeShore", "CAEN 1", "CAEN 2", "NI mod 2&3", "NI mod 1") -> (w844:bool[])
            n290 = call "check_ups.vi"() -> ("Error: no voltages read"=w828:bool, "Timestamp last measured"=→"Timestamp last \nmeasured (UPS)":timestamp, "Minimum input voltage measured"=w838:dbl)  [unwired: 8 in, 1 out]
            "Minimum input voltage measured" <- w838
            n291 = property on="Det.P input #" class="DigNum (strict)"() -> ("Value"=w864:i32)  [unwired: 2 in, 2 out]
            n292 = Or Array Elements(Boolean array=w849) -> (logical OR=→"Comm. status":bool)
            n293 = for {
              tunnel: w849 -> [w885] mode=indexing
              tunnel: w844 -> [w884] mode=indexing
              tunnel: [w883] -> w843 mode=indexing
              n294 = And(x=w885, y=w884) -> (x .and. y?=w883:bool)
            }
            n295 = Index Array(array=w865, index=w864) -> (element=w861:dbl)
            n296 = Less?(x=w838, y="UPS Voltage \nLower Threshold") -> (x < y?=w830:bool)
            n297 = Equal?(x=w838, y=-1.0) -> (x = y?=w829:bool)
            n298 = Less?(x=w861, y="Underpressure threshold") -> (x < y?=w859:bool)
            n299 = Build Array(w830, w829, w828) -> (w827:bool[])
            n300 = Or Array Elements(Boolean array=w843) -> (logical OR=w833:bool)
            n301 = Greater?(x=w861, y="Overpressure threshold") -> (0:w860:bool)
            n302 = Or(x=w860, y=w859) -> (x .or. y?=w858:bool)
            "Det. P. warning" <- w858
            n303 = Or Array Elements(Boolean array=w827) -> (logical OR=w826:bool)
            "Warning" <- w826
            n304 = And(x="UPS", y=w826) -> (x .and. y?=w832:bool)
            n305 = And(x=w858, y="Detector Pressure") -> (x .and. y?=w834:bool)
            n306 = local read "Det. T."() -> (w824:i32[])
            n307 = Build Array("T 1", "T 2", "T 3", "T 4", "T 5", "T 6") -> (w823:bool[])
            n308 = for {
              tunnel: w866 -> [w895]
              tunnel: w824 -> [w894] mode=indexing
              tunnel: w823 -> [w888] mode=indexing
              tunnel: [w887] -> w835 mode=indexing
              tunnel: [w886] -> w850 mode=indexing
              n309 = Index Array(array=w895, index=w894) -> (element=w891:dbl)
              n310 = Less?(x=w891, y="Low Temp threshold") -> (x < y?=w890:bool)
              n311 = Greater?(x=w891, y="High Temp threshold") -> (0:w889:bool)
              n312 = Or(x=w890, y=w889) -> (x .or. y?=w886:bool)
              n313 = And(x=w888, y=w886) -> (x .and. y?=w887:bool)
            }
            n314 = Index Array(array=w850) -> (element #1=→"Boolean":bool, element #2=→"Boolean 2":bool, element #3=→"Boolean 3":bool, element #4=→"Boolean 4":bool, element #5=→"Boolean 5":bool, element #6=→"Boolean 6":bool)  [unwired: 6 in]
            n315 = Build Array (concatenate)(w835, w834, w833, w832) -> (w831:bool[])
            n316 = Or Array Elements(Boolean array=w831) -> (logical OR=w825:bool)
            "Alarm state" <- w825
          }
          frame #8 {
            # "Testing alarm will not interfere"
            # "Act on alarm"
            n317 = Or(x="Test alarm", y=w902) -> (x .or. y?=w903:bool)
            n318 = case shown="True" w903 {
              tunnel: "Test alarm" -> [_ w909]
              tunnel: w900 -> [_ w917]
              tunnel: w899 -> [_ w916]
              tunnel: w898 -> [w906 w907]
              tunnel: "Alarm armed" -> [_ w914]
              tunnel: [w906 w908] -> w896
              frame False {
                # "Timer stays at previous value"
              }
              frame True {
                n319 = Get Date/Time In Seconds() -> (seconds since 1Jan1904=w921:timestamp)
                n320 = To Double Precision Float(number=w921) -> (double precision float=w918:dbl)
                n321 = Multiply(x="Repeat Alarm SMS\nevery N minutes", y=60.0) -> (x*y=w910:dbl)
                n322 = Subtract(x=w918, y=w907) -> (x-y=w913:dbl)
                n323 = Greater?(x=w913, y=w910) -> (0:w915:bool)
                n324 = And(x=w914, y=w915) -> (x .and. y?=w912:bool)
                n325 = Or(x=w909, y=w912) -> (x .or. y?=w911:bool)
                n326 = case shown="True" w911 {
                  tunnel: w909 -> [_ w928]
                  tunnel: w917 -> [_ w940]
                  tunnel: w916 -> [_ w923]
                  tunnel: [w922 w925] -> w908
                  tunnel: w907 -> [w922 w924]
                  frame False {
                    # "Alarm not armed, or defined time has not yet passed"
                  }
                  frame True {
                    # "Average T in Det."
                    n327 = local read "Det. T."() -> (w946:i32[])
                    n328 = local read "Det.P input #"() -> (w947:i32)
                    n329 = case shown="True" w928 {
                      tunnel: ["Error encountered inXAMS! Status:" "TESTING the XAMS alarm. Status:"] -> w939
                      tunnel: [w952 w955] -> w925
                      tunnel: w924 -> [_ w955]
                      frame False {
                        n330 = Get Date/Time In Seconds() -> (seconds since 1Jan1904=w953:timestamp)
                        n331 = To Double Precision Float(number=w953) -> (double precision float=w952:dbl)
                      }
                      frame True {
                      }
                    }
                    n332 = for {
                      tunnel: w923 -> [w966]
                      tunnel: w946 -> [w962] mode=indexing
                      tunnel: [w965] -> w945 mode=indexing
                      tunnel: [w963] -> w931 mode=indexing
                      n333 = Index Array(array=w966, index=w962) -> (element=w965:dbl)
                      n334 = Format Into String(format string="%.0f", w962) -> (resulting string=w959:string)  [unwired: 2 in, 1 out]
                      n335 = Format Into String(format string="%.3f", w965) -> (resulting string=w957:string)  [unwired: 2 in, 1 out]
                      n336 = Concatenate Strings("\nCh: " ("format string"), w959, ", Temp: " ("format string"), w957) -> (w963:string)
                    }
                    n337 = Index Array(array=w940, index=w947) -> (element=w941:dbl)
                    n338 = Array Size(array=w945) -> (size(s)=w943:i32)
                    n339 = Add Array Elements(numeric array=w945) -> (sum=w944:dbl)
                    n340 = Format Into String(format string="%.3f", w941) -> (resulting string=w935:string)  [unwired: 2 in, 1 out]
                    n341 = Divide(x=w944, y=w943) -> (x/y=w932:dbl)
                    n342 = Format Into String(format string="%.3f", w932) -> (resulting string=w929:string)  [unwired: 2 in, 1 out]
                    n343 = Format Date/Time String() -> (date/time string=w937:string)  [unwired: 3 in]
                    n344 = Concatenate Strings(w939, "\nDate/time: ", w937, "\nDetector Pressure: ", w935, "\nTemperatures (°C):", w931, "\nAverage detector temperature: ", w929) -> (w927:string)
                    n345 = for {
                      tunnel: w927 -> [w951]
                      tunnel: "Phone numbers" -> [w950] mode=indexing
                      n346 = call "send_sms.vi"("Message content"=w951, "Phone number"=w950) -> ("standard error"=→"standard error (SMS script)":string, "standard output"=→"Alarm (or test) message":string)  [unwired: 8 in]
                    }
                  }
                }
              }
            }
            n347 = And(x="Shut off heater \nif Alarm is active", y=w902) -> (x .and. y?=w904:bool)
            "Alarm active 2" <- "Alarm armed"
          }
          frame #9 {
            # "Daily e-mail"
            n348 = Get Date/Time In Seconds() -> (seconds since 1Jan1904=w977:timestamp)
            n349 = To Double Precision Float(number=w977) -> (double precision float=w976:dbl)
            n350 = Get Date/Time String(want seconds? (F)=FALSE) -> (time string=w979:string)  [unwired: 2 in, 1 out]
            n351 = Subtract(x=w976, y=w968) -> (x-y=w975:dbl)
            n352 = Equal?(x=w979, y="Send status email at time:") -> (x = y?=w972:bool)
            n353 = Greater?(x=w975, y=62) -> (0:w971:bool)
            n354 = Build Array("Send daily email?", w972, w971) -> (w970:bool[])
            n355 = And Array Elements(Boolean array=w970) -> (logical AND=w969:bool)
            n356 = case shown="True" w969 {
              tunnel: w983 -> [_ w1015]
              tunnel: w982 -> [_ w998]
              tunnel: w981 -> [_ w1007]
              tunnel: w968 -> [w984 _]
              tunnel: [w984 w993] -> w967
              frame False {
              }
              frame True {
                # "Average T in Det."
                n357 = local read "Det. T."() -> (w1016:i32[])
                n358 = Not Equal To 0?(x="Number of Bonus lines") -> (x != 0?=w986:bool)
                n359 = case shown="True" w986 {
                  tunnel: [w1021 w1024] -> w987
                  tunnel: "Number of Bonus lines" -> [_ w1027]
                  frame False {
                    n360 = Build Array("\n[Bonus line module inactive]") -> (w1021:string[])
                  }
                  frame True {
                    n361 = Build Path(base path=path "C:/Users/xams/Desktop/New XAMS Slow Control", name or relative path="cool_beans.txt") -> (appended path=w1028:path)
                    n362 = call-poly <vilib>:"Read Delimited Spreadsheet.vi"("file path (dialog if empty)"=w1028) -> ("all rows"=w1031:string[][])  [unwired: 9 in, 5 out]
                    n363 = Array Size(array=w1031) -> (size(s)=w1033:i32[])
                    n364 = Index Array(array=w1033) -> (element=w1032:i32)  [unwired: 1 in]
                    n365 = for {
                      N: w1027 -> [_]
                      tunnel: w1032 -> [w1038]
                      tunnel: w1031 -> [w1037]
                      tunnel: [w1034] -> w1025 mode=indexing
                      n366 = Random Number (0-1)() -> (number: 0 to 1=w1041:dbl)
                      n367 = Multiply(x=w1038, y=w1041) -> (x*y=w1040:dbl)
                      n368 = Round To Nearest(number=w1040) -> (nearest integer value=w1039:dbl)
                      n369 = Index Array(array=w1037, index (row)=w1039) -> (element=w1035:string[])  [unwired: 1 in]
                      n370 = Concatenate Strings("\n", w1035) -> (w1034:string)
                    }
                    n371 = Concatenate Strings("\n\nBy the way, did you know?", w1025) -> (w1023:string)
                    n372 = Build Array(w1023) -> (w1024:string[])
                  }
                }
                n373 = local read "Det.P input #"() -> (w1008:i32)
                n374 = for {
                  tunnel: w1016 -> [w1050] mode=indexing
                  tunnel: [w1051] -> w1000 mode=indexing
                  tunnel: w1015 -> [w1044]
                  tunnel: [w1043] -> w1014 mode=indexing
                  n375 = Index Array(array=w1044, index=w1050) -> (element=w1043:dbl)
                  n376 = Format Into String(format string="%.0f", w1050) -> (resulting string=w1047:string)  [unwired: 2 in, 1 out]
                  n377 = Format Into String(format string="%.2f", w1043) -> (resulting string=w1045:string)  [unwired: 2 in, 1 out]
                  n378 = Concatenate Strings("\nCh: " ("format string"), w1047, ", Temp: " ("format string"), w1045, "°C." ("format string")) -> (w1051:string)
                }
                n379 = Array Size(array=w1014) -> (size(s)=w1019:i32)
                n380 = Add Array Elements(numeric array=w1014) -> (sum=w1020:dbl)
                n381 = Index Array(array=w1007, index=w1008) -> (element=w1005:dbl)
                n382 = Divide(x=w1020, y=w1019) -> (x/y=w1017:dbl)
                n383 = Format Into String(format string="%.3f", w1005) -> (resulting string=w1003:string)  [unwired: 2 in, 1 out]
                n384 = Format Into String(format string="%.2f", w1017) -> (resulting string=w997:string)  [unwired: 2 in, 1 out]
                n385 = Select(t="ACTIVE!!!!!", s=w998, f="inactive.") -> (s? t:f=w1010:string)
                n386 = Concatenate Strings("Hello, XAMS teammembers.", "\n\nThe alarm is currently ", w1010, "\n\nThe latest detector pressure is: ", w1003, " bar." ("format string"), "\nTemperatures inside the detector are:", w1000, "\nThe average detector temperature is ", w997, "°C." ("format string"), "\n\nThank you for doing your best today, once again!\nRegards, SC.", w987) -> (w992:string)
                "Status email preview" <- w992
                n387 = call "custom_email_program.vi"("mail server"="smtp.nikhef.nl", "return address"="return address", "message"=w992, "subject ([No Subject])"="XAMS daily status email.", "Email Adresses"="Email Adresses") -> ()  [unwired: 6 in, 1 out]
                n388 = Get Date/Time In Seconds() -> (seconds since 1Jan1904=w994:timestamp)
                n389 = To Double Precision Float(number=w994) -> (double precision float=w993:dbl)
              }
            }
          }
        }
        n390 = Decrement(x="Cycles to execute") -> (x-1=w248:dbl)
        n391 = Decrement(x=w248) -> (x-1=w247:dbl)
        n392 = Greater?(x=w231, y=w247) -> ()  [unwired: 1 out]
        n393 = Decrement(x="Clear data every N cycles") -> (x-1=w228:dbl)
        n394 = Greater?(x=w231, y=w228) -> (0:w230:bool)
        n395 = And(x="Auto-clear data?", y=w230) -> (x .and. y?=w233:bool)
        n396 = Or(x=w233, y="Clear data") -> (x .or. y?=w235:bool)
        n397 = case shown="False" w235 {
          tunnel: w246 -> [w276 _]
          tunnel: [w276 dbl[][] []] -> w245
          tunnel: w244 -> [w275 _]
          tunnel: [w275 w282] -> w243
          tunnel: w242 -> [w274 _]
          tunnel: [w274 w282] -> w241
          tunnel: w240 -> [w273 _]
          tunnel: [w273 w280] -> w239
          tunnel: w238 -> [w272 _]
          tunnel: [w272 w278] -> w237
          tunnel: w231 -> [w271 _]
          tunnel: [w271 0] -> w232
          frame False {
          }
          frame True {
            w282 = 0.0
            n398 = Get Date/Time In Seconds() -> (seconds since 1Jan1904=w279:timestamp)
            n399 = To Double Precision Float(number=w279) -> (double precision float=w281:dbl)
            n400 = Build Array(w279) -> (w278:timestamp[])
            n401 = Build Array(w281, w281) -> (w280:dbl[])
          }
        }
        n402 = Or(x=FALSE, y="stop") -> (x .or. y?=w268:bool)
        "Auto-clear" <- "Auto-clear data?"
      }
    }
    frame True {
    }
  }
  n403 = flat-sequence {
    tunnel: w15 -> [w1088]
    tunnel: w11 -> [w1079]
    tunnel: w10 -> [w1076]
    tunnel: w9 -> [w1071]
    tunnel: w2 -> [w1060]
    frame #0 {
      w1084 = u16 2 items=["1"=1, "2"=2] ("Heater Output (1:1)")
      w1085 = u16 0 items=["Off", "Low (On)", "Medium", "High"] ("Range (0:Off)")
      # "Turn off heater, shutdown COM"
      # "Error Handling and Post-Processing (EHaPP)"
      n404 = Unbundle(w1088) -> ("VISA resource name out"=w1087:refnum<visa-resource-name>, "error out"=w1086:errorcluster)
      n405 = Unbundle(w1079) -> ("VISA resource name out"=w1078:refnum<visa-resource-name>, "error out"=w1077:errorcluster)
      n406 = Unbundle(w1076) -> ("VISA resource name out"=w1075:refnum<visa-resource-name>, "error out"=w1074:errorcluster)
      n407 = Unbundle(w1071) -> ("task out"=w1069:refnum<k21>, "error out"=w1067:errorcluster)
      n408 = Unbundle(w1060) -> ("task out"=w1064:refnum<k21>, "error out"=w1062:errorcluster)
      n409 = call <vilib>:"DAQmx Stop Task.vi"("task/channels in"=w1069, "error in"=w1067) -> ("task out"=w1068:refnum<k21>, "error out"=w1066:errorcluster)  [unwired: 12 in]
      n410 = call <vilib>:"DAQmx Stop Task.vi"("task/channels in"=w1064, "error in"=w1062) -> ("task out"=w1063:refnum<k21>, "error out"=w1061:errorcluster)  [unwired: 12 in]
      n411 = call <instrlib>:"Configure Output Range and Manual Value.vi"("VISA resource name"=w1087, "Heater Output (1:1)"=w1084, "Range (0:Off)"=w1085, "Manual Output (0.00 %)"=0.0, "error in (no error)"=w1086) -> ("VISA resource name out"=w1082:refnum<visa-resource-name>, "error out"=w1081:errorcluster)  [unwired: 9 in]
      n412 = call <instrlib>:"Close.vi"("error in (no error)"=w1077, "VISA resource name"=w1078) -> ("error out"=w1073:errorcluster)  [unwired: 9 in]
      n413 = call <instrlib>:"Close.vi"("error in (no error)"=w1074, "VISA resource name"=w1075) -> ("error out"=w1072:errorcluster)  [unwired: 9 in]
      n414 = call <instrlib>:"Close.vi"("error in (no error)"=w1081, "VISA resource name"=w1082) -> ("error out"=w1080:errorcluster)  [unwired: 9 in]
      n415 = call <vilib>:"DAQmx Clear Task.vi"("task in"=w1068, "error in"=w1066) -> ("error out"=w1070:errorcluster)  [unwired: 13 in]
      n416 = call <vilib>:"DAQmx Clear Task.vi"("task in"=w1063, "error in"=w1061) -> ("error out"=w1065:errorcluster)  [unwired: 13 in]
      n417 = call <vilib>:"Simple Error Handler.vi"("error in (no error)"=w1080) -> ()  [unwired: 4 in, 5 out]
      n418 = call <vilib>:"Simple Error Handler.vi"("error in (no error)"=w1073) -> ()  [unwired: 4 in, 5 out]
      n419 = call <vilib>:"Simple Error Handler.vi"("error in (no error)"=w1072) -> ()  [unwired: 4 in, 5 out]
      n420 = call <vilib>:"Simple Error Handler.vi"("error in (no error)"=w1070) -> ()  [unwired: 4 in, 5 out]
      n421 = call <vilib>:"Simple Error Handler.vi"("error in (no error)"=w1065) -> ()  [unwired: 4 in, 5 out]
    }
  }
  n422 = Array Size(array=w25) -> (size(s)=w28:i32)
  n423 = Decrement(x=w28) -> (x-1=w27:i32)
  n424 = Index Array(array=w25, index #1=w27, index #2=1 ("index")) -> (element #1=w26:timestamp, element #2=w7:timestamp)
  n425 = To Double Precision Float(number=w26) -> (double precision float=w24:dbl)
  n426 = To Double Precision Float(number=w7) -> (double precision float=w23:dbl)
  n427 = Subtract(x=w24, y=w23) -> ()  [unwired: 1 out]
  "Started up?" <- w19
